vi "Wide Field Drift Correction.vi"(7 "Calling VI Ref":refnum<vi>) -> ()   [LabVIEW 2020]
uses:
  Hardware Configuration/Hardware Configuration Controls/Device Type.ctl
  Hardware Configuration/Hardware Configuration Controls/Device Function.ctl
  WFDC Controls/WFDC Notifier Element.ctl
  WFDC Controls/WFDC Actions.ctl
  <vilib>/vision/Image Controls.llb/IMAQ Image.ctl
  WFDC Controls/WFDC External Sync.ctl
  WFDC Controls/WFDC Cycle Pause.ctl
  WFDC Controls/WFDC Status.ctl
  WFDC Controls/WFDC Default XY Stage Settings.ctl
  <vilib>/Utility/miscctls.llb/LVPointTypeDef.ctl
  Orca Flash Capture Manager/Orca Flash Capture Manager Controls/Orca Flash Capture Sync.ctl
  Device Library/Cameras/IDS/IDS Controls/IDS Actions.ctl
  Device Library/Cameras/IDS/IDS Controls/IDS Parameters.ctl
  Device Library/Cameras/IDS/IDS Controls/IDS Parameter List.ctl
  Device Library/Cameras/IDS/IDS Controls/IDS ROI.ctl
  Device Library/Cameras/IDS/IDS Controls/IDS IMAQ Key Info.ctl
  Device Library/Stages/Stages Controls/Stage Actions.ctl
  e645b282-29c8-4eda-9ede-5df860dd8c52.vi
panel:
  in  "Main Tab":T1(tab)
  out "Remote Start":bool
  out "Running":bool
  out "Z Drift (µm)":dbl=1.0 format="%.3g"
  out "Axis 2 Drift (Pixels)":dbl=1.0 format="%.3g"
  out "Axis 1 Drift (Pixels)":dbl=1.0 format="%.3g"
  out "Z Stage Position":dbl(graph)
  out "Z Drift Amount":dbl(graph)
  out "XY Drift Correction Active":bool
  out "Error":bool
  in  "Setup New":bool
  in  "Find Focus":bool
  in  "Smooth Points":i32=1
  in  "Smooth Z Data":bool
  in  "Z Step Correction Limit (µm)":dbl=1.0
  in  "Stage Defaults":bool
  in  "Invert Y Axis":bool
  in  "Invert X Axis":bool
  in  "Flip XY Axis":bool
  in  "Frame Accumulations":u16=20
  in  "Calibration Scan Range (µm)":dbl=1.0
  in  "Cycle Sync XY Correction":bool=TRUE
  in  "Track XY Drift":bool=TRUE
  in  "Correct XY Drift":bool=TRUE
  in  "XY Drift Threshold (pixels)":dbl=0.2
  in  "XY Drift Step (µm)":dbl=0.1
  in  "Z Position Offset (µm)":dbl
  in  "Z Drift Threshold (µm)":dbl=0.02
  in  "Correct Z Drift":bool=TRUE
  in  "Abort Capture If Error":bool=TRUE
  in  "Cycle Sync Z Correction":bool
  out "Z Stage":dbl=1.0 format="%.3g"
  out "Z Drift":dbl=1.0 format="%.3g"
  in  "CC Box Size":i32=11
  in  "Correction Limit":u8=50
  out "Correction Step":u8=1
  out "CC Fit":dbl[][](graph)
  out "CC Image":dbl[][](graph)
  in  "Abort Remote":bool
  in  "CC Cutoff":dbl=0.2
  in  "Roundness Cutoff":dbl=1.75
  out "Axis 1":dbl=1.0 format="%.3g"
  out "Axis 2":dbl=1.0 format="%.3g"
  out "XY Active":bool
  out "Z Active":bool
  out "Error Message":string
  out "Current Frame":u32=1
  in  "Capture":bool
  in  "Number of Frames":u32=1
  in  "Image Save Path":path
  in  "Exposure Time (ms)":dbl
  in  "Image Display":bool
  in  "Live Preview":bool
  in  "Quit":bool
  # "General Settings"
  # "XY Stage Settings"
  # "XY Drift Settings"
  # "Z Drift Settings"
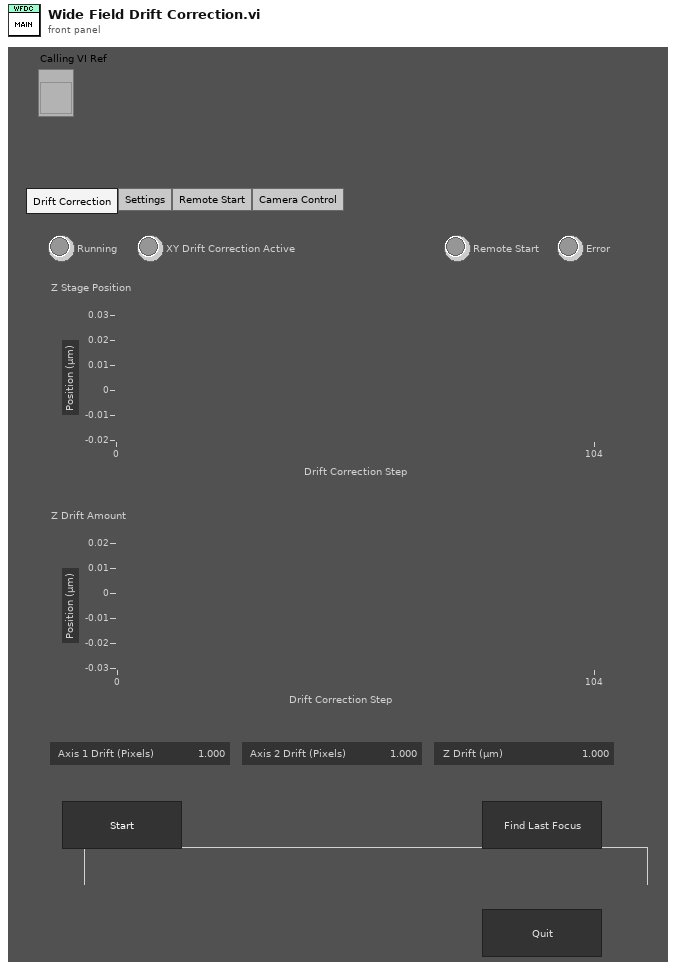
[diagram p1: front panel]
types:
  T1 = enum32{"Drift Correction", "Settings", "Remote Start", "Camera Control"}
  T2 = typedef "Orca Flash Capture Sync.ctl" = cluster{"Image Ref":T3, "Cycle Number":u16, "Camera Running?":bool, "Capture?":bool}
  T3 = typedef "IMAQ Image.ctl" = refnum<image>
  T4 = enum16{"Always On", "Always Off", "Off While Running"}
  T5 = typedef "LVPointTypeDef.ctl" = cluster{"Horizontal":i16, "Vertical":i16}
  T6 = typedef "WFDC Default XY Stage Settings.ctl" = cluster{"Flip XY":bool, "Invert X":bool, "Invert Y":bool}
  T7 = typedef "WFDC Cycle Pause.ctl" = enum16{"Pause Requested", "Paused", "Resume Requested", "Resumed"}
  T8 = typedef "WFDC Status.ctl" = enum16{"Idle", "Busy", "DC Active", "Error", "Canceled"}
  T9 = typedef "WFDC External Sync.ctl" = cluster{"Cycle Sync":T7, "Z Offset":dbl, "WFDC Status":T8}
  T10 = typedef "WFDC Actions.ctl" = enum16{"Error Check", "Remote Start", "Move to Pos", "Pre Start Get Drift", "Pre Start Check Drift", "Pre Start Z Drift", "Pre Start XY Drift", "Pre Start ReFocus", "Setup New DC", "Setup Camera", "Get Ref Images", "Calc Calibration", "Switch Tabs", "Get Drift", "Z Drift", "XY Drift", "Start Cycle", "Stop DC", "Abort Remote", "Exit Loop", "Set Error", "Generate Calibration", "Quit"}
  T11 = typedef "WFDC Notifier Element.ctl" = cluster{"WFDC Actions":T10, "Initial XYZ Positions":dbl[], "Ref Images":T3[], "Calibration (slope, inter)":dbl[], "Base Path":path, "Latest Scan Path":path, "Error":errorcluster, "XYZ Drift":dbl[]}
  T12 = typedef "Device Function.ctl" = enum16{"Primary", "Secondary", "Overview", "Wide Field Drift Correction", "642 nm Excitation", "560 nm Excitation", "940 nm Excitation", "546 nm Excitation", "488 nm Excitation", "405 nm Excitation", "Objective Drift Correction", "4Pi Objective Lock", "Objective XY", "Objective Z", "Sample XY", "Sample Coarse Z", "Sample Z", "4Pi Lower", "4Pi Upper", "Mojo", "Adj Cavity", "Line Scanning", "Alert"}
  T13 = typedef "Device Type.ctl" = enum16{"AOTF", "Camera", "Deformable Mirror", "Laser", "Microscope Base", "Shutter", "Stage", "Waveform", "FPGA", "Email", "Filter Wheel", "Spinning Disk"}
  T14 = typedef "LVRectTypeDef.ctl" = cluster{"Left":i16, "Top":i16, "Right":i16, "Bottom":i16}
  T15 = typedef "LVBoundsTypeDef.ctl" = cluster{"Width":u32, "Height":u32}
  T16 = enum8{"Enabled", "Disabled", "Disabled and Grayed Out"}
  T17 = typedef "IDS Actions.ctl" = enum16{"Error Check", "Initialize", "Preview", "Record", "Abort", "Record Settings", "Set Parameter", "Get Parameter", "Set ROI", "Get ROI", "Status", "Quit"}
  T18 = typedef "IDS Parameter List.ctl" = enum16{"Exposure Time (s)", "Binning"}
  T19 = typedef "IDS Parameters.ctl" = cluster{"Parameter":T18, "Value":dbl}
  T20 = typedef "IDS ROI.ctl" = cluster{"H Offset":i32, "V Offset":i32, "H Width":i32, "V Width":i32}
  T21 = typedef "IDS IMAQ Key Info.ctl" = cluster{"Frame":u32, "Sensor Height":i32, "Sensor Width":i32, "ROI Height":i32, "ROI Width":i32, "ROI Enable?":bool, "Bit per Pixel":u8}
  T22 = typedef "Stage Actions.ctl" = enum16{"Get Position", "MVR", "MOVE", "HALT", "ONTARGET", "ERROR", "REFERENCE", "INIT", "VELOCITY", "STATUS", "EXIT", "HOME", "ZEROPOS", "NANOPOS", "ANALOG", "QUIT"}
  T23 = enum32{"Page Enabled", "Page Disabled", "Page Disabled & Grayed"}
  T24 = typedef "2D Gaussian - Best Fit Parameters.ctl" = cluster{"Amplitude":dbl, "X Position":dbl, "Y Position":dbl, "X Width":dbl, "Y Width":dbl, "Offset":dbl}
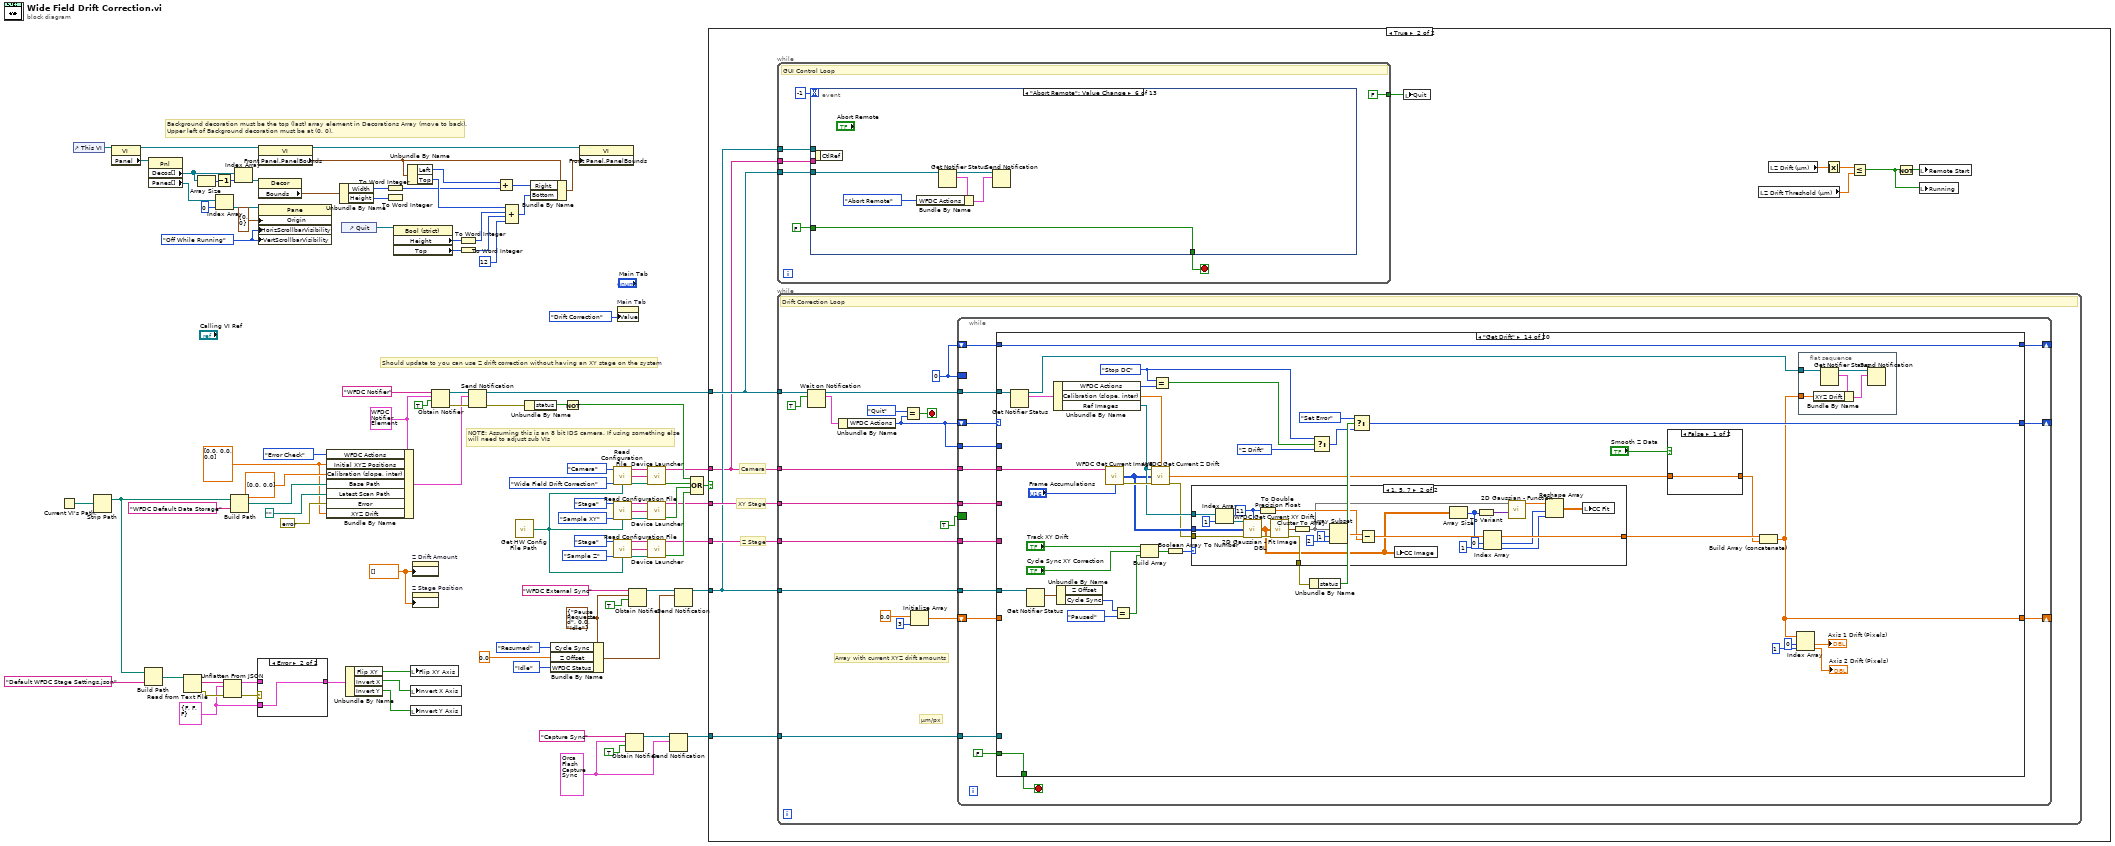
[diagram p0: block diagram]
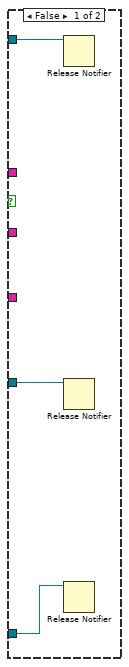
[diagram p3: hidden frame]
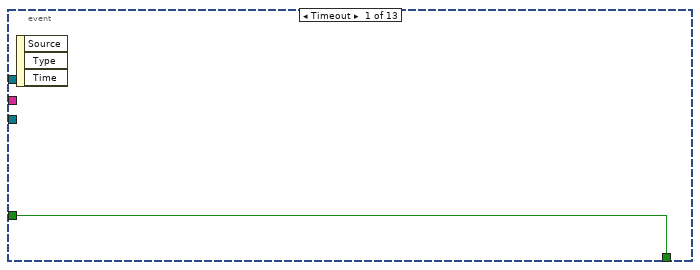
[diagram p4: hidden frame]
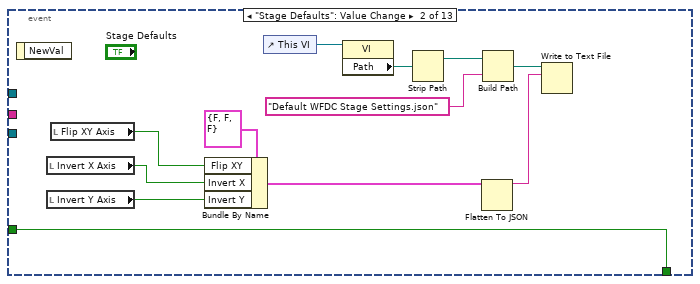
[diagram p5: hidden frame]
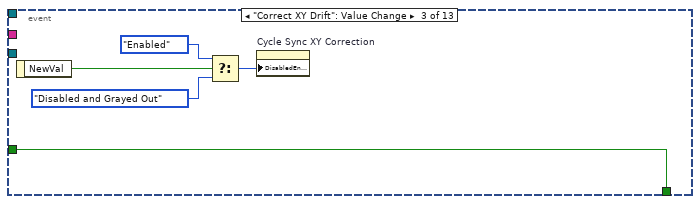
[diagram p6: hidden frame]
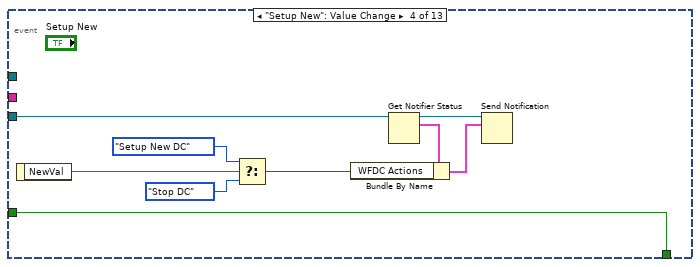
[diagram p7: hidden frame]
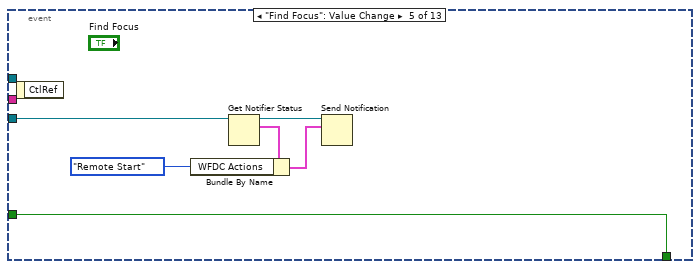
[diagram p8: hidden frame]
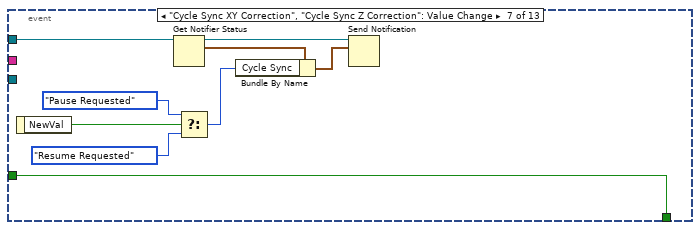
[diagram p9: hidden frame]
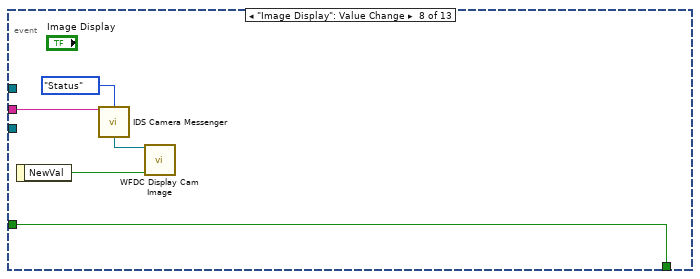
[diagram p10: hidden frame]
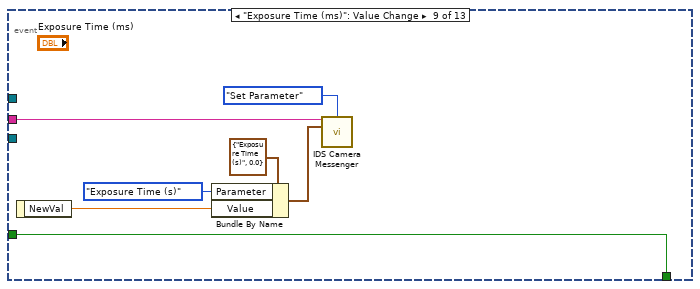
[diagram p11: hidden frame]
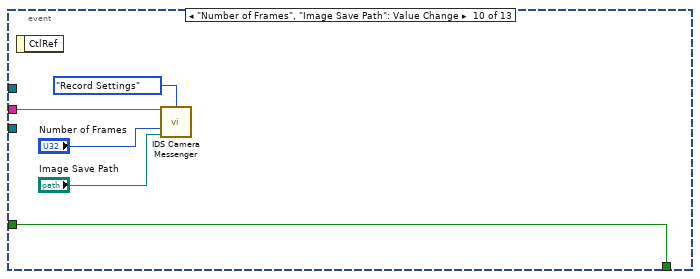
[diagram p12: hidden frame]
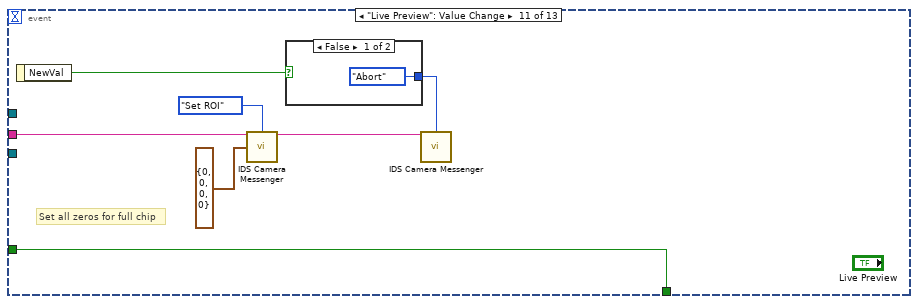
[diagram p13: hidden frame]
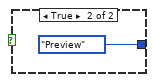
[diagram p14: hidden frame]
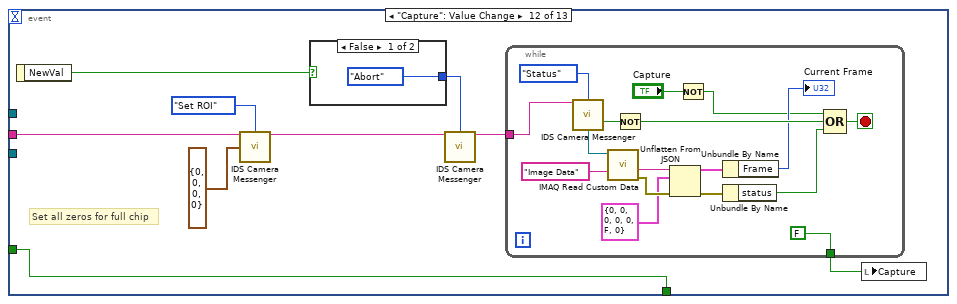
[diagram p15: hidden frame]
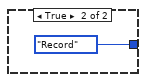
[diagram p16: hidden frame]
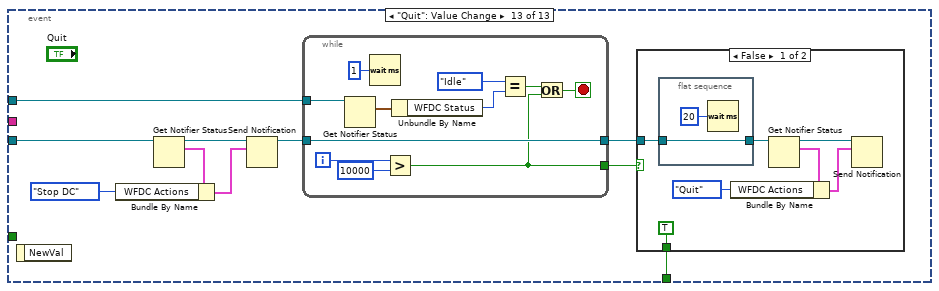
[diagram p17: hidden frame]
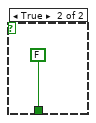
[diagram p18: hidden frame]
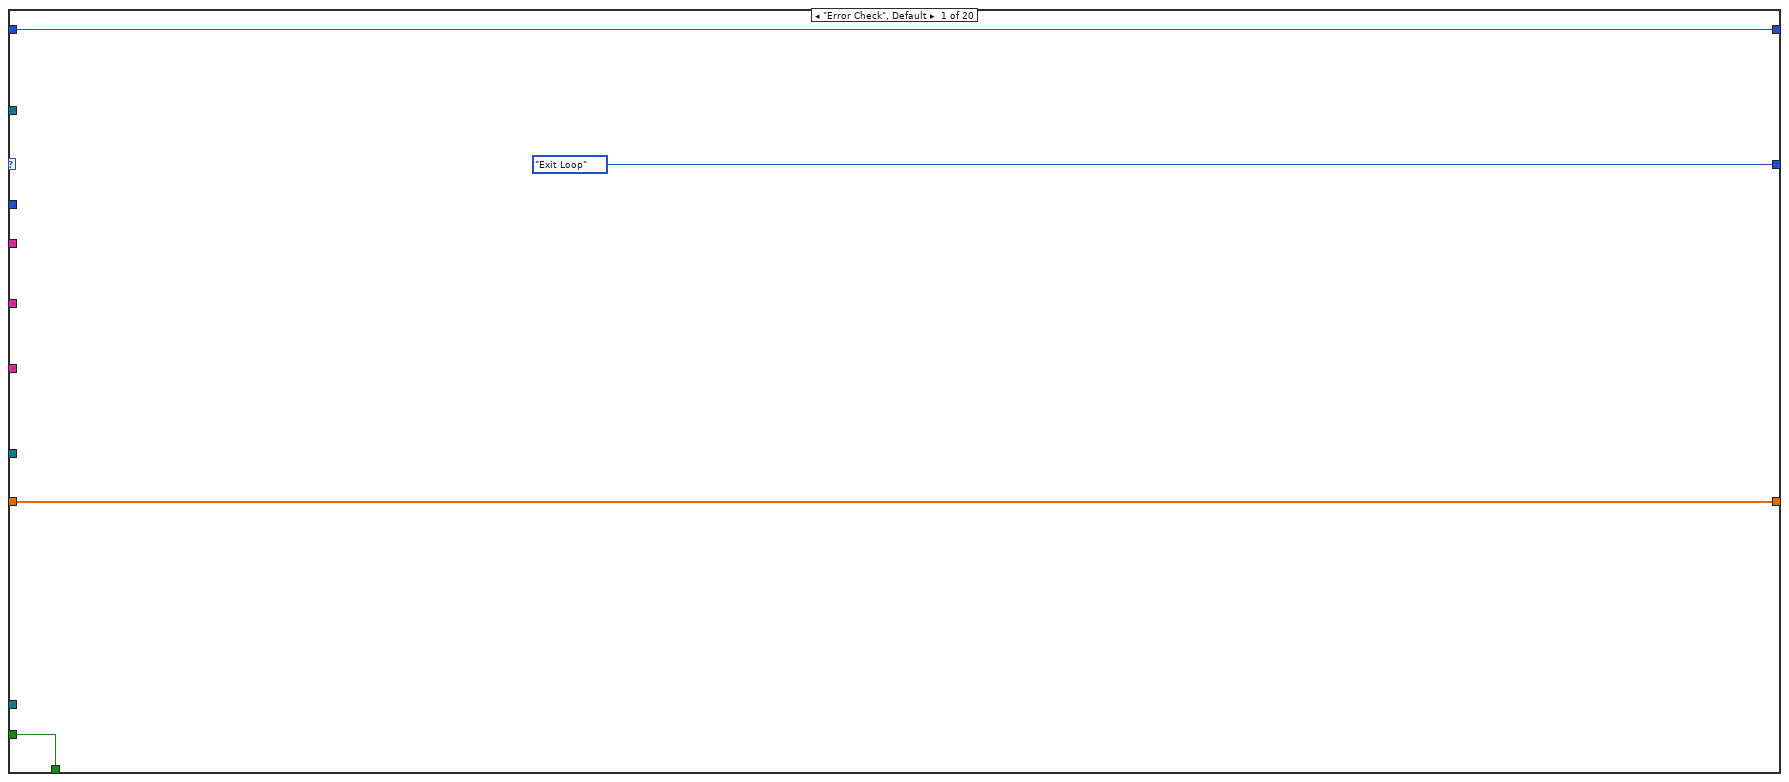
[diagram p19: hidden frame]
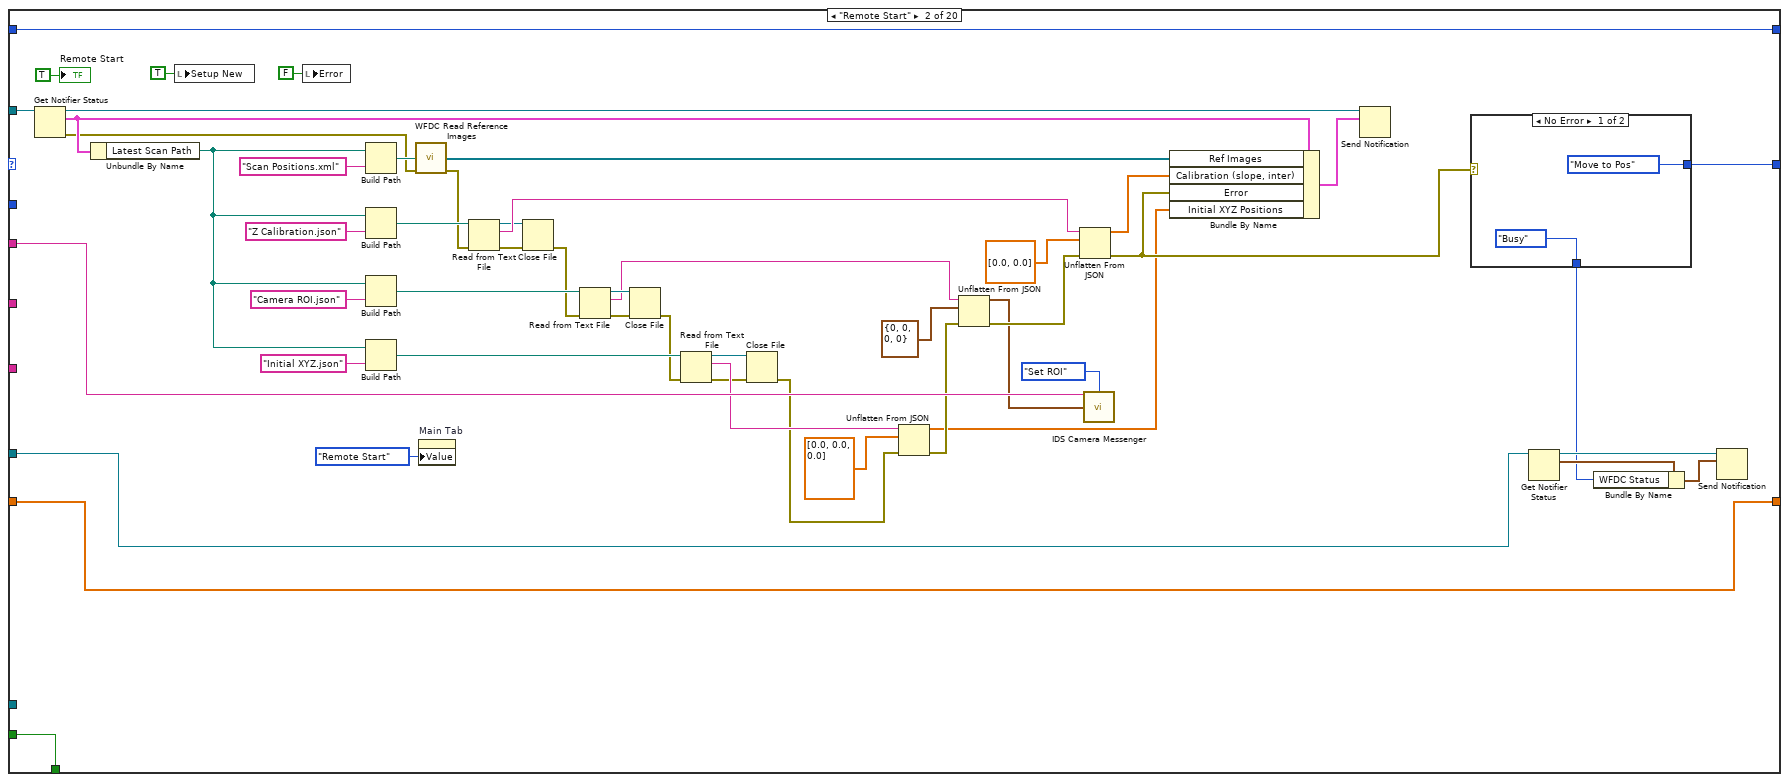
[diagram p20: hidden frame]
diagram:
  w2 = T2 {"Image Ref"=refnum, "Cycle Number"=0, "Camera Running?"=FALSE, "Capture?"=FALSE} ("Capture Sync Data")
  w17 = T4."Off While Running" ("Vertical Scrollbar Visibility")
  w39 = T6 {"Flip XY"=FALSE, "Invert X"=FALSE, "Invert Y"=FALSE} ("Default WFDC Stage Settings")
  w56 = T9 {"Cycle Sync"=enum."Pause Requested", "Z Offset"=0.0, "WFDC Status"=enum."Idle"} ("WFDC External Sync")
  w1 = dbl[] [0.0, 0.0, 0.0] ("Initial XYZ Positions")
  w65 = dbl[] []
  w67 = T11 {"WFDC Actions"=enum."Error Check", "Initial XYZ Positions"=[], "Ref Images"=[], "Calibration (slope, inter)"=[], "Base Path"=path "", "Latest Scan Path"=path "", "Error"={"status"=FALSE, "code"=0, "source"=""}, "XYZ Drift"=[]} ("WFDC Notifier Element")
  # "Background decoration must be the top (last) array element in Decorations Array (move to back).\nUpper left of Background decoration must be at (0, 0)."
  # "Should update to you can use Z drift correction without having an XY stage on the system"
  # "NOTE: Assuming this is an 8 bit IDS camera. If using something else\nwill need to adjust sub VIs"
  n1 = Current VI's Path() -> (path=w4:path)
  n2 = control-ref of="This VI"() -> (w9:refnum<vi>)
  n3 = Strip Path(path=w4) -> (stripped path=w3:path)  [unwired: 1 out]
  n4 = property class="VI"(reference=w9) -> (reference out=w18:refnum<vi>, "Panel"=w10:refnum<vi>)  [unwired: 1 in, 1 out]
  n5 = Build Path(base path=w3, name or relative path="Default WFDC Stage Settings.json") -> (appended path=w44:path)
  n6 = property class="Pnl"(reference=w10) -> ("Decos[]"=w8:refnum<vi>[], "Panes[]"=w14:refnum<vi>[])  [unwired: 1 in, 2 out]
  n7 = Read from Text File(file (use dialog)=w44) -> (text=w43:string, error out=w42:errorcluster)  [unwired: 3 in, 2 out]
  n8 = Array Size(array=w8) -> (size(s)=w6:i32)
  n9 = Decrement(x=w6) -> (x-1=w7:i32)
  n10 = Index Array(array=w14, index=0) -> (element=w13:refnum<vi>)
  n11 = Unflatten From JSON(JSON string=w43, type and defaults=w39, error in (no error)=w42) -> (value=w40:T6, error out=w41:errorcluster)  [unwired: 4 in]
  n12 = Build Path(base path=w3, name or relative path="WFDC Default Data Storage") -> (appended path=w59:path)
  n13 = Index Array(array=w8, index=w7) -> (element=w16:refnum<vi>)
  n14 = case shown="Error" w41 {
    tunnel: w40 -> [w99 _]
    tunnel: [w99 w100] -> w38
    tunnel: w39 -> [_ w100]
    frame No Error {
    }
    frame Error {
    }
  }
  n15 = property class="VI"(reference=w18) -> (reference out=w20:refnum<vi>, "Front Panel.PanelBounds"=w21:T14)  [unwired: 1 in, 1 out]
  n16 = property class="Decor"(reference=w16) -> ("Bounds"=w19:T15)  [unwired: 1 in, 2 out]
  n17 = property class="Pane"(reference=w13, "Origin"=T5 {"Horizontal"=0, "Vertical"=0}, "HorizScrollbarVisibility"=w17, "VertScrollbarVisibility"=w17) -> ()  [unwired: 1 in, 2 out]
  n18 = Bundle By Name(cluster=w67, "WFDC Actions"=WFDC_Actions."Error Check", "Initial XYZ Positions"=w1, "Calibration (slope, inter)"=dbl[] [0.0, 0.0], "Base Path"=w59, "Latest Scan Path"=path "", "Error"=errorcluster {"status"=FALSE, "code"=0, "source"=""}, "XYZ Drift"=w1) -> (w66:T11)
  n19 = Unbundle By Name(w19) -> ("Width"=w24:u32, "Height"=w27:u32)
  n20 = control-ref of="Quit"() -> (w11:refnum<vi>)
  n21 = Unbundle By Name(w38) -> ("Flip XY"=w37:bool, "Invert X"=w36:bool, "Invert Y"=w35:bool)
  n22 = To Word Integer(number=w24) -> (16bit integer=w26:i16)
  n23 = To Word Integer(number=w27) -> ()  [unwired: 1 out]
  n24 = property class="Bool (strict)"(reference=w11) -> ("Height"=w29:u32, "Top"=w30:i32)  [unwired: 1 in, 2 out]
  n25 = Unbundle By Name(w21) -> ("Left"=w23:i16, "Top"=w34:i16)
  n26 = local write "Flip XY Axis"(w37) -> ()
  n27 = local write "Invert X Axis"(w36) -> ()
  n28 = local write "Invert Y Axis"(w35) -> ()
  n29 = property on="Z Drift Amount" class="WFChart (strict)"("History Data"=w65) -> ()  [unwired: 2 in, 2 out]
  n30 = property on="Z Stage Position" class="WFChart (strict)"("History Data"=w65) -> ()  [unwired: 2 in, 2 out]
  n31 = Obtain Notifier(name (unnamed)="WFDC Notifier", notification data type=w67, create if not found? (T)=TRUE) -> (notifier out=w81:refnum<notifier>, error out=w79:errorcluster)  [unwired: 1 in, 1 out]
  n32 = To Word Integer(number=w29) -> (16bit integer=w32:i16)
  n33 = To Word Integer(number=w30) -> (16bit integer=w33:i16)
  n34 = Send Notification(notification=w66, notifier=w81, error in (no error)=w79) -> (notifier out=w80:refnum<notifier>, error out=w74:errorcluster)
  n35 = Add(x=w23, y=w26) -> (x+y=w25:i16)
  n36 = Compound Arithmetic op=ADD(w34, w32, w33, i16 12 ("y")) -> (w28:i16)
  n37 = call "Get HW Config File Path.vi"() -> ("File Path"=w63:path)  [unwired: 14 in, 1 out]
  n38 = Unbundle By Name(w74) -> ("status"=w73:bool)
  n39 = Bundle By Name(cluster=w21, "Right"=w25, "Bottom"=w28) -> (w22:T14)
  n40 = Bundle By Name(cluster=w56, "Cycle Sync"=WFDC_Cycle_Pause."Resumed", "Z Offset"=0.0, "WFDC Status"=WFDC_Status."Idle") -> (w50:T9)
  n41 = Not(x=w73) -> (.not. x?=w72:bool)
  n42 = property class="VI"(reference=w20, "Front Panel.PanelBounds"=w22) -> ()  [unwired: 1 in, 2 out]
  n43 = call "Read Configuration File.vi"("Device Type"=Device_Type."Camera", "Device Function"=Device_Function."Wide Field Drift Correction", "Config File Path"=w63) -> ("Unique Notifier Name"=w97:string, "Device Ports/IDs/Channels"=w96:string[], "Device Engine Path"=w95:path)  [unwired: 9 in, 1 out]
  n44 = call "Read Configuration File.vi"("Device Type"=Device_Type."Stage", "Device Function"=Device_Function."Sample XY", "Config File Path"=w63) -> ("Unique Notifier Name"=w88:string, "Device Ports/IDs/Channels"=w89:string[], "Device Engine Path"=w90:path)  [unwired: 9 in, 1 out]
  n45 = call "Read Configuration File.vi"("Device Type"=Device_Type."Stage", "Device Function"=Device_Function."Sample Z", "Config File Path"=w63) -> ("Unique Notifier Name"=w87:string, "Device Ports/IDs/Channels"=w86:string[], "Device Engine Path"=w85:path)  [unwired: 9 in, 1 out]
  n46 = property on="Main Tab" class="TabCtl (strict)"("Value"=T1."Drift Correction" ("Main Tab")) -> ()  [unwired: 2 in, 2 out]
  n47 = Obtain Notifier(name (unnamed)="Capture Sync", notification data type=w2, create if not found? (T)=TRUE) -> (notifier out=w47:refnum<notifier>)  [unwired: 1 in, 2 out]
  n48 = Obtain Notifier(name (unnamed)="WFDC External Sync", notification data type=w56, create if not found? (T)=TRUE) -> (notifier out=w52:refnum<notifier>)  [unwired: 1 in, 2 out]
  n49 = call "Device Launcher.vi"("Notifier Name"=w97, "Device Ports/IDs/Channels"=w96, "Device Engine Path"=w95) -> ("Notifier Name"=w70:string, "Running?"=w77:bool)  [unwired: 11 in]
  n50 = call "Device Launcher.vi"("Notifier Name"=w88, "Device Ports/IDs/Channels"=w89, "Device Engine Path"=w90) -> ("Notifier Name"=w69:string, "Running?"=w76:bool)  [unwired: 11 in]
  n51 = call "Device Launcher.vi"("Notifier Name"=w87, "Device Ports/IDs/Channels"=w86, "Device Engine Path"=w85) -> ("Notifier Name"=w68:string, "Running?"=w75:bool)  [unwired: 11 in]
  n52 = Send Notification(notification=w2, notifier=w47) -> (notifier out=w46:refnum<notifier>)  [unwired: 1 in, 1 out]
  n53 = Send Notification(notification=w50, notifier=w52) -> (notifier out=w51:refnum<notifier>)  [unwired: 1 in, 1 out]
  n54 = Compound Arithmetic op=OR(w72, w77, w76, w75) -> (w71:bool)
  n55 = case shown="True" w71 {
    tunnel: w80 -> [w103 w113]
    tunnel: w70 -> [_ w109]
    tunnel: w69 -> [_ w115]
    tunnel: w68 -> [_ w114]
    tunnel: w51 -> [w102 w111]
    tunnel: w46 -> [w101 w110]
    frame False {
      n56 = Release Notifier(notifier=w103) -> ()  [unwired: 2 in, 3 out]
      n57 = Release Notifier(notifier=w102) -> ()  [unwired: 2 in, 3 out]
      n58 = Release Notifier(notifier=w101) -> ()  [unwired: 2 in, 3 out]
    }
    frame True {
      # "Z Stage"
      # "XY Stage"
      # "Camera"
      n59 = while {
        tunnel: w113 -> [w272]
        tunnel: w109 -> [w264]
        tunnel: w115 -> [w267]
        tunnel: w114 -> [w266]
        tunnel: w111 -> [w259]
        tunnel: w110 -> [w258]
        stop <- w268 stop-if-true
        w256 = u8 0
        # "µm/px"
        # "Array with current XYZ drift amounts"
        # "Drift Correction Loop"
        n60 = Wait on Notification(notifier=w272, ignore previous (F)=TRUE) -> (notifier out=w271:refnum<notifier>, notification=w270:T11)  [unwired: 2 in, 2 out]
        n61 = Unbundle By Name(w270) -> ("WFDC Actions"=w265:T10)
        n62 = Equal?(x=WFDC_Actions."Quit", y=w265) -> (x = y?=w268:bool)
        n63 = Initialize Array(0.0 ("element"), 3 ("dimension size")) -> (w262:dbl[])
        n64 = while {
          tunnel: w271 -> [w279]
          shift-right: [w283] -> _
          shift-left: w265 -> [w287]
          tunnel: w264 -> [w286]
          tunnel: w267 -> [w285]
          tunnel: w266 -> [w284]
          tunnel: w265 -> [w280]
          tunnel: w259 -> [w278]
          shift-right: [w276] -> _
          shift-left: w262 -> [w277]
          tunnel: w258 -> [w275]
          border: TRUE -> [_]
          border: w256 -> [_]
          shift-right: [w273] -> _
          shift-left: w256 -> [w274]
          stop <- w281 stop-if-true
          n65 = case shown="\"Get Drift\"" w287 {
            selector: w287 -> [_ _ _ _ _ _ _ _ _ _ _ _ _ _ _ _ _ w1001 _ _]
            tunnel: w286 -> [_ w327 w373 w421 _ _ _ w577 _ w662 w706 w737 _ w813 _ _ _ w1013 _ _]
            tunnel: w285 -> [_ _ w360 _ _ _ w559 _ _ _ w699 _ _ _ _ w913 _ _ _ _]
            tunnel: w284 -> [_ _ w372 _ _ w484 _ w576 _ _ w696 _ _ _ w863 _ _ _ _ _]
            tunnel: [WFDC_Actions."Exit Loop" ("x") w321 WFDC_Actions."Pre Start Get Drift" ("f") w409 w454 w486 w556 w581 w641 w670 WFDC_Actions."Calc Calibration" ("x") w712 WFDC_Actions."Get Drift" ("x") w788 w852 w905 WFDC_Actions."Get Drift" ("x") WFDC_Actions."Exit Loop" ("x") WFDC_Actions."Exit Loop" ("x") WFDC_Actions."Quit" ("x")] -> w283
            tunnel: FALSE -> [w291 w343 w375 w423 w473 w489 w560 w585 w642 w672 w707 w741 w769 w815 w884 w914 w965 w1014 _ _]
            tunnel: [w291 w343 w375 w423 w473 w489 w560 w585 w642 w672 w707 w741 w769 w815 w884 w914 w965 w1014 TRUE TRUE] -> w281
            tunnel: w280 -> [_ _ _ _ _ _ _ _ w634 _ _ w714 _ _ _ _ _ _ _ _]
            tunnel: w279 -> [_ w342 w368 w422 _ w487 _ w579 _ w666 w705 w740 _ w814 w885 _ _ w1010 _ w1028]
            tunnel: w278 -> [_ w312 w353 _ _ _ _ _ w636 w658 _ w727 w758 w811 w867 w907 w963 w1003 _ w1027]
            tunnel: w277 -> [w289 w313 w369 _ w464 w477 w558 w575 w640 w668 w686 w735 w776 _ w870 w899 w966 w1008 w1019 w1026]
            tunnel: [w289 w313 w369 w408 w464 w477 w558 w575 w640 w668 w686 w735 w776 w778 w870 w899 w966 w1008 w1019 w1026] -> w276
            tunnel: w275 -> [_ _ _ _ _ _ _ _ _ _ _ _ _ _ _ _ w962 _ _ w1023]
            tunnel: w274 -> [w288 w292 w348 w379 w451 w474 w523 _ w631 w656 w678 w708 w756 w781 w851 w897 w959 w989 w1017 w1022]
            tunnel: [w288 w292 w348 w379 w450 w474 w523 u8 0 w631 w656 w678 w708 w756 w781 w851 w897 w959 w989 w1017 w1022] -> w273
            frame "Error Check", Default {
            }
            frame "Remote Start" {
              n66 = Get Notifier Status(notifier=w342) -> (notifier out=w334:refnum<notifier>, current notification=w337:T11, error out=w322:errorcluster)  [unwired: 1 in, 2 out]
              n67 = Unbundle By Name(w337) -> ("Latest Scan Path"=w314:path)
              n68 = local write "Setup New"(TRUE ("Setup New")) -> ()
              n69 = local write "Error"(FALSE ("Error")) -> ()
              n70 = Build Path(base path=w314, name or relative path="Scan Positions.xml") -> (appended path=w340:path)
              n71 = Build Path(base path=w314, name or relative path="Z Calibration.json") -> (appended path=w333:path)
              n72 = Build Path(base path=w314, name or relative path="Camera ROI.json") -> (appended path=w325:path)
              n73 = Build Path(base path=w314, name or relative path="Initial XYZ.json") -> (appended path=w311:path)
              n74 = call "WFDC Read Reference Images.vi"("Scan Positions File Path"=w340, "Error"=w322) -> ("Ref Images"=w336:T3[], "Error"=w329:errorcluster)  [unwired: 12 in]
              n75 = property on="Main Tab" class="TabCtl (strict)"("Value"=T1."Remote Start" ("Main Tab")) -> ()  [unwired: 2 in, 2 out]
              n76 = Read from Text File(file (use dialog)=w333, error in=w329) -> (refnum out=w308:refnum<file>, text=w332:string, error out=w304:errorcluster)  [unwired: 2 in, 1 out]
              n77 = Close File(refnum=w308, error in=w304) -> (error out=w301:errorcluster)  [unwired: 1 out]
              n78 = Read from Text File(file (use dialog)=w325, error in=w301) -> (refnum out=w307:refnum<file>, text=w302:string, error out=w303:errorcluster)  [unwired: 2 in, 1 out]
              n79 = Close File(refnum=w307, error in=w303) -> (error out=w298:errorcluster)  [unwired: 1 out]
              n80 = Read from Text File(file (use dialog)=w311, error in=w298) -> (refnum out=w306:refnum<file>, text=w309:string, error out=w305:errorcluster)  [unwired: 2 in, 1 out]
              n81 = Close File(refnum=w306, error in=w305) -> (error out=w299:errorcluster)  [unwired: 1 out]
              n82 = Unflatten From JSON(JSON string=w309, type and defaults=dbl[] [0.0, 0.0, 0.0], error in (no error)=w299) -> (value=w297:dbl[], error out=w300:errorcluster)  [unwired: 4 in]
              n83 = Unflatten From JSON(JSON string=w302, type and defaults=T20 {"H Offset"=0, "V Offset"=0, "H Width"=0, "V Width"=0} ("ROI Setup"), error in (no error)=w300) -> (value=w323:T20, error out=w324:errorcluster)  [unwired: 4 in]
              n84 = Unflatten From JSON(JSON string=w332, type and defaults=dbl[] [0.0, 0.0], error in (no error)=w324) -> (value=w330:dbl[], error out=w320:errorcluster)  [unwired: 4 in]
              n85 = call "IDS Camera Messenger.vi"("Notifier Name"=w327, "IDS Actions"=IDS_Actions."Set ROI", "ROI Setup"=w323) -> ()  [unwired: 7 in, 6 out]
              n86 = Bundle By Name(cluster=w337, "Ref Images"=w336, "Calibration (slope, inter)"=w330, "Error"=w320, "Initial XYZ Positions"=w297) -> (w335:T11)
              n87 = Send Notification(notification=w335, notifier=w334) -> ()  [unwired: 1 in, 2 out]
              n88 = case shown="No Error" w320 {
                tunnel: [WFDC_Actions."Move to Pos" ("x") WFDC_Actions."Exit Loop" ("x")] -> w321
                tunnel: [WFDC_Status."Busy" ("WFDC Status") WFDC_Status."Error" ("WFDC Status")] -> w317
                frame No Error {
                }
                frame Error {
                }
              }
              n89 = Get Notifier Status(notifier=w312) -> (notifier out=w319:refnum<notifier>, current notification=w318:T9)  [unwired: 1 in, 3 out]
              n90 = Bundle By Name(cluster=w318, "WFDC Status"=w317) -> (w316:T9)
              n91 = Send Notification(notification=w316, notifier=w319) -> ()  [unwired: 1 in, 2 out]
              "Remote Start" <- TRUE ("Remote Start")
            }
            frame "Move to Pos" {
              n92 = Get Notifier Status(notifier=w368) -> (current notification=w367:T11)  [unwired: 1 in, 4 out]
              n93 = Unbundle By Name(w367) -> ("Ref Images"=w366:T3[], "Initial XYZ Positions"=w359:dbl[])
              n94 = Get Notifier Status(notifier=w353) -> (notifier out=w356:refnum<notifier>, current notification=w355:T9)  [unwired: 1 in, 3 out]
              n95 = call "IDS Camera Messenger.vi"("Notifier Name"=w373, "IDS Actions"=IDS_Actions."Preview") -> ()  [unwired: 8 in, 6 out]
              n96 = Bundle By Name(cluster=w355, "WFDC Status"=WFDC_Status."Busy") -> (w354:T9)
              n97 = Split 1D Array(array=w359, index=2) -> (first subarray=w357:dbl[], second subarray=w350:dbl[])
              n98 = Send Notification(notification=w354, notifier=w356) -> ()  [unwired: 1 in, 2 out]
              n99 = Index Array(array=w366, index=1) -> ()  [unwired: 1 out]
              n100 = call "Stages Messenger.vi"("Stage Notifier Name"=w360, "Actions"=Stage_Actions."MOVE", "Setpoint"=w357, "Axis"=bool[] [TRUE, TRUE], "Exit While Busy?"=FALSE) -> ()  [unwired: 7 in, 4 out]
              n101 = call "Stages Messenger.vi"("Stage Notifier Name"=w372, "Actions"=Stage_Actions."MOVE", "Setpoint"=w350, "Axis"=bool[] [TRUE], "Exit While Busy?"=FALSE) -> ("Stage Notifier Name (Dup)"=w352:string)  [unwired: 7 in, 3 out]
              n102 = flat-sequence {
                tunnel: w352 -> [w377]
                tunnel: [w377] -> _
                frame #0 {
                  n103 = Wait (ms)(milliseconds to wait=u32 350) -> ()  [unwired: 1 out]
                }
              }
            }
            frame "Pre Start Get Drift" {
              w410 = WFDC_Actions."Abort Remote" ("x")
              n104 = Get Notifier Status(notifier=w422) -> (current notification=w420:T11)  [unwired: 1 in, 4 out]
              n105 = Unbundle By Name(w420) -> ("WFDC Actions"=w415:T10, "Initial XYZ Positions"=w378:dbl[], "Calibration (slope, inter)"=w385:dbl[], "Ref Images"=w418:T3[])
              n106 = call "WFDC Get Current Image.vi"("IDS Camera Notifier Name"=w421, "Frames"=u16 10) -> ("Image - U16"=w417:u16[][], "Error"=w419:errorcluster)  [unwired: 11 in, 1 out]
              n107 = call "WFDC Get Current Z Drift.vi"("Ref Images"=w418, "Z Calibration (slope, inter)"=w385, "Current Image"=w417, "Error In"=w419) -> ("Z Position (µm)"=w384:dbl, "Error Out"=w416:errorcluster)  [unwired: 10 in]
              n108 = Index Array(array=w418, index=1) -> (element=w403:T3)
              n109 = Index Array(array=w378, index=2) -> (element=w386:dbl)
              n110 = Subtract(x=w386, y=w384) -> (x-y=w383:dbl)
              n111 = feedback #1() -> (w394:bool)
              n112 = Select(t=35 ("hBox"), s=w394, f="CC Box Size") -> (s? t:f=w396:i32)
              n113 = call "WFDC Get Current XY Drift.vi"("Center Ref Image"=w403, "hBox"=w396, "Current Image"=w417, "Error In"=w416) -> ("Drift (px)"=w393:dbl[], "Corr Array"=w392:dbl[][], "Error Out"=w395:errorcluster)  [unwired: 9 in]
              "CC Image" <- w392
              n114 = Absolute Value(x=w393) -> (abs(x)=w381:dbl[])
              n115 = Greater?(x=w381, y=5.0) -> (0:w399:bool[])
              n116 = Or Array Elements(Boolean array=w399) -> (logical OR=w398:bool)
              n117 = feedback-in #1(w398) -> ()
              n118 = case shown="True" w394 {
                tunnel: w393 -> [_ w447]
                tunnel: w392 -> [w426 w449]
                tunnel: [w427 w446] -> w390
                tunnel: [w442 w449] -> w391
                tunnel: w395 -> [w434 w448]
                tunnel: [w431 w448] -> w389
                tunnel: w396 -> [w429 _]
                frame False {
                  n119 = To Double Precision Float(number=w429) -> (double precision float=w428:dbl)
                  n120 = Array Size(array=w426) -> (size(s)=w439:i32[])
                  n121 = call "2D Gaussian - Fit Image DBL.vi"("Image In (DBL)"=w426, "Error In"=w434) -> ("Best Fit Params"=w445:T24, "Error Out"=w433:errorcluster)  [unwired: 12 in]
                  n122 = To Variant(anything=w439) -> (Variant=w441:variant)
                  n123 = Cluster To Array(cluster=w445) -> (array=w432:dbl[])
                  n124 = Index Array(array=w439, index #1=0 ("index"), index #2=1 ("index")) -> (element #1=w438:i32, element #2=w437:i32)
                  n125 = call "2D Gaussian - Function.vi"("data"=w441, "a"=w432) -> ("f(X,a)"=w440:dbl[])  [unwired: 2 in, 2 out]
                  n126 = call "WFDC Check CC Errors.vi"("Fit Result"=w432, "CC Image"=w426, "Contrast Limit"="CC Cutoff", "Roundness Limit"="Roundness Cutoff", "Error In"=w433) -> ("Error Out"=w431:errorcluster)  [unwired: 10 in]
                  n127 = Array Subset(array=w432, index=1, length=2) -> (w430:dbl[])
                  n128 = Reshape Array(w440, w438, w437) -> (w442:dbl[][])
                  n129 = Subtract(x=w430, y=w428) -> (x-y=w427:dbl[])
                }
                frame True {
                  n130 = Reverse 1D Array(array=w447) -> (reversed array=w446:dbl[])
                }
              }
              "CC Fit" <- w391
              n131 = Unbundle By Name(w389) -> ("source"=→"Error Message":string, "status"=w388:bool)
              n132 = Build Array (concatenate)(w390, w383) -> (w408:dbl[])
              n133 = Index Array(array=w408, index #1=0 ("index"), index #2=1 ("index")) -> (element #1=→"Axis 1":dbl, element #2=→"Axis 2":dbl)
              n134 = Equal?(x=w410, y=w415) -> (x = y?=w412:bool)
              n135 = Select(t=w410, s=w412, f=WFDC_Actions."Pre Start Check Drift" ("x")) -> (s? t:f=w411:T10)
              n136 = Select(t=WFDC_Actions."Set Error" ("x"), s=w388, f=w411) -> (s? t:f=w409:T10)
            }
            frame "Pre Start Check Drift" {
              n137 = Increment(x=w451) -> (x+1=w450:u8)
              "Correction Step" <- w450
              n138 = local read "Z Drift Threshold (µm)"() -> (w461:dbl)
              n139 = local read "XY Drift Threshold (pixels)"() -> (w466:dbl)
              n140 = Index Array(array=w464, index=2) -> (element=w462:dbl)
              n141 = Array Subset(array=w464, index=0, length=2) -> (w467:dbl[])
              n142 = Absolute Value(x=w462) -> (abs(x)=w453:dbl)
              n143 = Absolute Value(x=w467) -> (abs(x)=w452:dbl[])
              n144 = Greater?(x=w453, y=w461) -> (0:w459:bool)
              n145 = Greater?(x=w452, y=w466) -> (0:w465:bool[])
              n146 = Or Array Elements(Boolean array=w465) -> (logical OR=w460:bool)
              n147 = Or(x=w460, y=w459) -> (x .or. y?=w458:bool)
              n148 = Greater?(x=w450, y="Correction Limit") -> (0:w457:bool)
              n149 = Select(t=WFDC_Actions."Pre Start Z Drift" ("x"), s=w458, f=WFDC_Actions."Switch Tabs") -> (s? t:f=w455:T10)
              n150 = Select(t=WFDC_Actions."Pre Start ReFocus" ("f"), s=w457, f=w455) -> (s? t:f=w454:T10)
            }
            frame "Pre Start Z Drift" {
              n151 = Get Notifier Status(notifier=w487) -> (current notification=w488:T11)  [unwired: 1 in, 4 out]
              n152 = Unbundle By Name(w488) -> ("WFDC Actions"=w485:T10)
              n153 = local write "XY Active"(FALSE ("XY Active")) -> ()
              n154 = Array Subset(array=w477, index=0, length=2) -> (w482:dbl[])
              n155 = Absolute Value(x=w482) -> (abs(x)=w481:dbl[])
              n156 = Greater?(x=w481, y=5.0) -> (0:w478:bool[])
              n157 = Or Array Elements(Boolean array=w478) -> (logical OR=w476:bool)
              n158 = case shown="False" w476 {
                tunnel: [w504 WFDC_Actions."Pre Start XY Drift" ("x")] -> w486
                tunnel: w485 -> [w503 _]
                tunnel: w477 -> [w501 _]
                tunnel: w484 -> [w497 _]
                frame False {
                  w505 = WFDC_Actions."Abort Remote" ("x")
                  n159 = local read "Z Drift Threshold (µm)"() -> (w499:dbl)
                  n160 = Index Array(array=w501, index=2) -> (element=w491:dbl)
                  "Z Drift" <- w491
                  n161 = Absolute Value(x=w491) -> (abs(x)=w500:dbl)
                  n162 = Greater?(x=w500, y=w499) -> (0:w498:bool)
                  n163 = case shown="True" w498 {
                    tunnel: w497 -> [w512 w521]
                    tunnel: w491 -> [_ w518]
                    tunnel: [w510 w515] -> w496
                    tunnel: [w511 w514] -> w494
                    frame False {
                      n164 = call "Stages Messenger.vi"("Stage Notifier Name"=w512, "Actions"=Stage_Actions."Get Position") -> ("Positions"=w511:dbl[], "Error"=w510:errorcluster)  [unwired: 10 in, 2 out]
                    }
                    frame True {
                      n165 = Build Array(w518) -> (w520:dbl[])
                      n166 = call "Stages Messenger.vi"("Stage Notifier Name"=w521, "Actions"=Stage_Actions."MVR", "Setpoint"=w520, "Axis"=bool[] [TRUE], "Exit While Busy?"=FALSE) -> ("Positions"=w514:dbl[], "Error"=w515:errorcluster)  [unwired: 7 in, 2 out]
                    }
                  }
                  n167 = Unbundle By Name(w496) -> ("status"=w495:bool)
                  n168 = Index Array(array=w494, index=0) -> (element=→"Z Stage":dbl)
                  n169 = Equal?(x=w505, y=w503) -> (x = y?=w507:bool)
                  n170 = Select(t=w505, s=w507, f=WFDC_Actions."Pre Start XY Drift" ("x")) -> (s? t:f=w506:T10)
                  n171 = Select(t=WFDC_Actions."Set Error" ("x"), s=w495, f=w506) -> (s? t:f=w504:T10)
                  "Z Active" <- TRUE ("Z Active")
                }
                frame True {
                }
              }
            }
            frame "Pre Start XY Drift" {
              n172 = local read "CC Box Size"() -> (w547:i32)
              n173 = local write "Z Active"(FALSE ("Z Active")) -> ()
              n174 = Array Subset(array=w558, index=0, length=2) -> (w525:dbl[])
              n175 = To Double Precision Float(number=w547) -> (double precision float=w546:dbl)
              n176 = Absolute Value(x=w525) -> (abs(x)=w541:dbl[])
              n177 = Subtract(x=w546, y=3.0) -> ()  [unwired: 1 out]
              n178 = Greater?(x=w541, y=5.0) -> (0:w545:bool[])
              n179 = local read "Flip XY Axis"() -> (w537:bool)
              n180 = local read "XY Drift Step (µm)"() -> (w528:dbl)
              n181 = local read "XY Drift Threshold (pixels)"() -> (w531:dbl)
              n182 = Or Array Elements(Boolean array=w545) -> (logical OR=w529:bool)
              n183 = Select(t=0.5, s=w529, f=w528) -> (s? t:f=w527:dbl)
              n184 = Absolute Value(x=w525) -> (abs(x)=w532:dbl[])
              n185 = Greater?(x=w532, y=w531) -> (0:w530:bool[])
              n186 = case shown="True" w537 {
                tunnel: w530 -> [w562 w566]
                tunnel: [w562 w565] -> w550
                tunnel: w525 -> [w561 w564]
                tunnel: [w561 w563] -> w535
                frame False {
                }
                frame True {
                  n187 = Reverse 1D Array(array=w564) -> (reversed array=w563:dbl[])
                  n188 = Reverse 1D Array(array=w566) -> (reversed array=w565:bool[])
                }
              }
              n189 = Greater?(x=w535, y=0.0) -> (0:w534:bool[])
              n190 = local read "Invert X Axis"() -> (w539:bool)
              n191 = local read "Invert Y Axis"() -> (w540:bool)
              n192 = Build Array(w539, w540) -> (w538:bool[])
              n193 = for {
                N: 2 -> [_]
                tunnel: [w571] -> w549 mode=indexing
                tunnel: w527 -> [w569]
                tunnel: w538 -> [w572] mode=indexing
                tunnel: w534 -> [w567] mode=indexing
                n194 = Negate(x=w569) -> (-x=w570:dbl)
                n195 = Select(t=w569, s=w567, f=w570) -> (s? t:f=w568:dbl)
                n196 = Negate(x=w568) -> (-x=w573:dbl)
                n197 = Select(t=w568, s=w572, f=w573) -> (s? t:f=w571:dbl)
              }
              n198 = call "Stages Messenger.vi"("Stage Notifier Name"=w559, "Actions"=Stage_Actions."MVR", "Setpoint"=w549, "Axis"=w550, "Exit While Busy?"=FALSE) -> ("Error"=w544:errorcluster)  [unwired: 7 in, 3 out]
              n199 = Select(t=WFDC_Actions."Set Error" ("x"), s=w544, f=WFDC_Actions."Pre Start Get Drift" ("x")) -> (s? t:f=w556:T10)
              "XY Active" <- TRUE ("XY Active")
            }
            frame "Pre Start ReFocus" {
              n200 = Get Notifier Status(notifier=w579) -> (current notification=w580:T11)  [unwired: 1 in, 4 out]
              n201 = feedback #2() -> (w583:u8)
              n202 = Increment(x=w583) -> (x+1=w584:u8)
              n203 = feedback-in #2(w584) -> ()
              n204 = Unbundle By Name(w580) -> ("Ref Images"=w578:T3[])
              n205 = Greater Than 0?(x=w583) -> (x > 0?=w582:bool)
              n206 = case shown="False" w582 {
                tunnel: [w591 WFDC_Actions."Abort Remote" ("x")] -> w581
                tunnel: w578 -> [w599 _]
                tunnel: w577 -> [w596 _]
                tunnel: w576 -> [w590 _]
                frame False {
                  n207 = Build Array(-20.0 ("element")) -> (w595:dbl[])
                  n208 = call "Stages Messenger.vi"("Stage Notifier Name"=w590, "Actions"=Stage_Actions."MVR", "Setpoint"=w595, "Axis"=bool[] [TRUE], "Exit While Busy?"=FALSE) -> ("Stage Notifier Name (Dup)"=w588:string)  [unwired: 7 in, 3 out]
                  n209 = call "Stall Data Flow.vim"("value in"=w588, "milliseconds to wait"=u32 300) -> ("value out"=w587:string)  [unwired: 1 out]
                  n210 = Index Array(array=w599, index=1) -> (element=w597:T3)
                  n211 = call "WFDC Scan Focus.vi"("Ref Image"=w597, "Camera Notifier"=w596, "Z Stage Notifier"=w587, "No. of Steps"=40, "Step Size (µm)"=1.0) -> ("Z Stage Notifier (Dup)"=w602:string, "Pos vs. Corr"=w601:dbl[][], "Canceled?"=w600:bool)  [unwired: 8 in]
                  n212 = case shown="True" w600 {
                    tunnel: w602 -> [w607 _]
                    tunnel: w601 -> [w606 _]
                    tunnel: [WFDC_Actions."Pre Start Get Drift" ("f") WFDC_Actions."Abort Remote" ("f")] -> w591
                    frame False {
                      n213 = Index Array(array=w606, index (col) #1=0 ("disabled index (col)"), index (col) #2=1 ("index (col)")) -> (element #1=w609:dbl[], element #2=w610:dbl[])  [unwired: 2 in]
                      n214 = disable-structure shown="Enabled" {
                        disable-tunnel: w610 -> [w616 w620]
                        disable-tunnel: w609 -> [w615 w621]
                        disable-tunnel: [w613 w617] -> w608
                        frame Enabled {
                          n215 = Array Max & Min(array=w616) -> (max index (indices)=w614:i32)  [unwired: 3 out]
                          n216 = Index Array(array=w615, index=w614) -> (element=w613:dbl)
                        }
                        frame Disabled {
                          n217 = call "1D Gaussian Fitting.vi"("X Values"=w621, "Y Values"=w620) -> ("Best Fit Parameters"=w619:dbl[])  [unwired: 11 in, 2 out]
                          n218 = Index Array(array=w619, index=1) -> (element=w617:dbl)
                        }
                      }
                      n219 = flat-sequence {
                        tunnel: w607 -> [w624]
                        tunnel: w608 -> [w623]
                        frame #0 {
                          n220 = Build Array(w623) -> (w622:dbl[])
                          n221 = call "Stages Messenger.vi"("Stage Notifier Name"=w624, "Actions"=Stage_Actions."MOVE", "Setpoint"=w622, "Axis"=bool[] [TRUE], "Exit While Busy?"=FALSE) -> ()  [unwired: 7 in, 4 out]
                        }
                        frame #1 {
                          n222 = Wait (ms)(milliseconds to wait=u32 350) -> ()  [unwired: 1 out]
                        }
                      }
                    }
                    frame True {
                    }
                  }
                }
                frame True {
                }
              }
            }
            frame "Setup New DC", "Generate Calibration" {
              n223 = case shown="\"Generate Calibration\", Default" w634 {
                tunnel: [WFDC_Actions."Setup Camera" ("f") w646] -> w641
                frame "Generate Calibration", Default {
                }
                frame "Setup New DC" {
                  n224 = Two Button Dialog(message="Is the Z stage is near its center position?", 1:"No" ("F button name (\"Cancel\")"), 2:"Yes" ("T button name (\"OK\")")) -> (T button?=w649:bool)
                  n225 = case shown="False" w649 {
                    selector: w649 -> [w653 w655]
                    tunnel: "Center Z Stage and start again" ("message") -> [w654 _]
                    tunnel: [w653 w655] -> w644
                    frame False {
                      n226 = One Button Dialog(message=w654) -> ()  [unwired: 1 in, 1 out]
                    }
                    frame True {
                    }
                  }
                  n227 = Select(t=WFDC_Actions."Setup Camera" ("x"), s=w644, f=WFDC_Actions."Exit Loop") -> (s? t:f=w646:T10)
                }
              }
              n228 = Get Notifier Status(notifier=w636) -> (notifier out=w638:refnum<notifier>, current notification=w637:T9)  [unwired: 1 in, 3 out]
              n229 = Bundle By Name(cluster=w637, "WFDC Status"=WFDC_Status."Busy") -> (w639:T9)
              n230 = local write "Error"(FALSE ("Error")) -> ()
              n231 = Send Notification(notification=w639, notifier=w638) -> ()  [unwired: 1 in, 2 out]
              "Running" <- TRUE ("Running")
            }
            frame "Setup Camera" {
              w669 = dbl[] []
              # "Set exposure time and select camera ROI"
              n232 = Get Notifier Status(notifier=w666) -> (notifier out=w667:refnum<notifier>, current notification=w665:T11)  [unwired: 1 in, 3 out]
              n233 = Unbundle By Name(w665) -> ("Base Path"=w661:path)
              n234 = property on="Z Drift Amount" class="WFChart (strict)"("History Data"=w669) -> ()  [unwired: 2 in, 2 out]
              n235 = property on="Z Stage Position" class="WFChart (strict)"("History Data"=w669) -> ()  [unwired: 2 in, 2 out]
              n236 = call "WFDC Setup Camera.vi"("Base Data Path"=w661, "Camera Notifier Name"=w662, "ROI File Name"="Camera ROI.json" ("name or relative path")) -> ("Current Save Path"=w663:path, "Canceled?"=w657:bool)  [unwired: 9 in, 2 out]
              n237 = Bundle By Name(cluster=w665, "Latest Scan Path"=w663) -> (w664:T11)
              n238 = Send Notification(notification=w664, notifier=w667) -> ()  [unwired: 1 in, 2 out]
              n239 = case shown="False" w657 {
                tunnel: w658 -> [_ w673]
                frame False {
                }
                frame True {
                  n240 = Get Notifier Status(notifier=w673) -> (notifier out=w676:refnum<notifier>, current notification=w675:T9)  [unwired: 1 in, 3 out]
                  n241 = Bundle By Name(cluster=w675, "WFDC Status"=WFDC_Status."Canceled") -> (w677:T9)
                  n242 = Send Notification(notification=w677, notifier=w676) -> ()  [unwired: 1 in, 2 out]
                }
              }
              n243 = Select(t=WFDC_Actions."Exit Loop", s=w657, f=WFDC_Actions."Get Ref Images" ("y")) -> (s? t:f=w670:T10)
            }
            frame "Get Ref Images" {
              n244 = call "Stages Messenger.vi"("Stage Notifier Name"=w699, "Actions"=Stage_Actions."Get Position") -> ("Positions"=w691:dbl[])  [unwired: 10 in, 3 out]
              n245 = call "Stages Messenger.vi"("Stage Notifier Name"=w696, "Actions"=Stage_Actions."Get Position") -> ("Stage Notifier Name (Dup)"=w695:string, "Positions"=w694:dbl[])  [unwired: 10 in, 2 out]
              n246 = Index Array(array=w691, index #1=0 ("index"), index #2=1 ("index")) -> (element #1=w689:dbl, element #2=w688:dbl)
              n247 = Index Array(array=w694, index=0) -> (element=w687:dbl)
              n248 = Get Notifier Status(notifier=w705) -> (notifier out=w703:refnum<notifier>, current notification=w702:T11)  [unwired: 1 in, 3 out]
              n249 = Unbundle By Name(w702) -> ("Latest Scan Path"=w682:path)
              n250 = Build Array(w689, w688, w687) -> (w683:dbl[])
              n251 = call "WFDC Get Reference Images.vi"("IDS Camera Notifier"=w706, "Data Save Path"=w682, "Z Stage Notifier"=w695, "Scan Range"="Calibration Scan Range (µm)", "Frame per Step"=u32 20, "Scan Positions File Name"="Scan Positions.xml" ("name or relative path")) -> ()  [unwired: 10 in]
              n252 = Build Path(base path=w682, name or relative path="Initial XYZ.json") -> (appended path=w680:path)
              n253 = Flatten To JSON(anything=w683) -> (JSON string=w679:string)  [unwired: 2 in, 1 out]
              n254 = Bundle By Name(cluster=w702, "Initial XYZ Positions"=w683) -> (w701:T11)
              n255 = Write to Text File(file (use dialog)=w680, text=w679) -> ()  [unwired: 2 in, 3 out]
              n256 = Send Notification(notification=w701, notifier=w703) -> ()  [unwired: 1 in, 2 out]
            }
            frame "Calc Calibration" {
              n257 = local read "Cycle Sync XY Correction"() -> (w726:bool)
              n258 = local read "Cycle Sync Z Correction"() -> (w725:bool)
              n259 = Get Notifier Status(notifier=w740) -> (notifier out=w711:refnum<notifier>, current notification=w739:T11)  [unwired: 1 in, 3 out]
              n260 = flat-sequence {
                tunnel: w739 -> [w755]
                tunnel: [w753] -> w738
                tunnel: w737 -> [w750]
                tunnel: [w750] -> w736
                tunnel: [w748] -> w728
                tunnel: w727 -> [w748]
                tunnel: [w746] -> w722
                tunnel: [w745] -> w723
                tunnel: w716 -> [w744]
                frame #0 {
                  n261 = Unbundle By Name(w755) -> ("Latest Scan Path"=w746:path)
                  n262 = call "WFDC Compute Z Calibration.vi"("Scan Positions File Name"="Scan Positions.xml" ("name or relative path"), "User Close?"=w744, "Data Path"=w746) -> ("Fit Slope"=w754:dbl, "Fit Intercept"=w752:dbl, "Ref Images"=w749:T3[], "Error"=w751:errorcluster)  [unwired: 9 in]
                  n263 = Build Array(w754, w752) -> (w745:dbl[])
                  n264 = Bundle By Name(cluster=w755, "Calibration (slope, inter)"=w745, "Error"=w751, "Ref Images"=w749) -> (w753:T11)
                }
              }
              n265 = Or(x=w726, y=w725) -> (x .or. y?=w724:bool)
              n266 = Equal?(x=WFDC_Actions."Generate Calibration", y=w714) -> (x = y?=w710:bool)
              n267 = Equal?(x=WFDC_Actions."Setup New DC", y=w714) -> (x = y?=w716:bool)
              n268 = Select(t=WFDC_Cycle_Pause."Pause Requested" ("Cycle Sync"), s=w724, f=WFDC_Cycle_Pause."Resumed" ("Cycle Sync")) -> (s? t:f=w730:T7)
              n269 = Get Notifier Status(notifier=w728) -> (notifier out=w734:refnum<notifier>, current notification=w733:T9)  [unwired: 1 in, 3 out]
              n270 = Bundle By Name(cluster=w733, "Cycle Sync"=w730) -> (w732:T9)
              n271 = Send Notification(notification=w732, notifier=w734) -> ()  [unwired: 1 in, 2 out]
              n272 = Send Notification(notification=w738, notifier=w711) -> ()  [unwired: 1 in, 2 out]
              n273 = Flatten To JSON(anything=w723) -> (JSON string=w719:string)  [unwired: 2 in, 1 out]
              n274 = Build Path(base path=w722, name or relative path="Z Calibration.json") -> (appended path=w720:path)
              n275 = Write to Text File(file (use dialog)=w720, text=w719) -> (refnum out=w718:refnum<file>)  [unwired: 2 in, 2 out]
              n276 = Close File(refnum=w718) -> ()  [unwired: 1 in, 2 out]
              n277 = case shown="True" w710 {
                tunnel: w736 -> [w743 _]
                frame False {
                  # "Start Camera"
                  n278 = call "IDS Camera Messenger.vi"("Notifier Name"=w743, "IDS Actions"=IDS_Actions."Preview") -> ()  [unwired: 8 in, 6 out]
                }
                frame True {
                }
              }
              n279 = Select(t=WFDC_Actions."Stop DC", s=w710, f=WFDC_Actions."Switch Tabs" ("x")) -> (s? t:f=w712:T10)
            }
            frame "Switch Tabs" {
              w757 = FALSE ("Z Active")
              n280 = local read "Cycle Sync XY Correction"() -> (w768:bool)
              n281 = local read "Cycle Sync Z Correction"() -> (w767:bool)
              n282 = local write "Z Active"(w757) -> ()
              n283 = local write "XY Active"(w757) -> ()
              n284 = local write "Remote Start"(w757) -> ()
              n285 = property on="Main Tab" class="TabCtl (strict)"("Value"=T1."Drift Correction" ("Main Tab")) -> ("Pages"=w773:refnum<vi>[])  [unwired: 2 in, 2 out]
              n286 = Or(x=w768, y=w767) -> (x .or. y?=w766:bool)
              n287 = Index Array(array=w773, index=3) -> (element=w771:refnum<vi>)
              n288 = property class="Page"(reference=w771, "PageEnb"=T23."Page Disabled & Grayed" ("Page Enabled State")) -> ()  [unwired: 1 in, 2 out]
              n289 = Select(t=WFDC_Cycle_Pause."Pause Requested" ("Cycle Sync"), s=w766, f=WFDC_Cycle_Pause."Resume Requested" ("Cycle Sync")) -> (s? t:f=w765:T7)
              n290 = Get Notifier Status(notifier=w758) -> (notifier out=w762:refnum<notifier>, current notification=w763:T9)  [unwired: 1 in, 3 out]
              n291 = Bundle By Name(cluster=w763, "WFDC Status"=WFDC_Status."DC Active", "Cycle Sync"=w765) -> (w764:T9)
              n292 = Send Notification(notification=w764, notifier=w762) -> ()  [unwired: 1 in, 2 out]
            }
            frame "Get Drift" {
              w789 = WFDC_Actions."Stop DC" ("x")
              n293 = Get Notifier Status(notifier=w814) -> (notifier out=w777:refnum<notifier>, current notification=w779:T11)  [unwired: 1 in, 3 out]
              n294 = Get Notifier Status(notifier=w811) -> (current notification=w810:T9)  [unwired: 1 in, 4 out]
              n295 = Unbundle By Name(w779) -> ("WFDC Actions"=w795:T10, "Calibration (slope, inter)"=w807:dbl[], "Ref Images"=w800:T3[])
              n296 = Unbundle By Name(w810) -> ("Cycle Sync"=w808:T7)  [unwired: 1 out]
              n297 = call "WFDC Get Current Image.vi"("IDS Camera Notifier Name"=w813, "Frames"="Frame Accumulations") -> ("Image - U16"=w799:u16[][], "Error"=w806:errorcluster)  [unwired: 11 in, 1 out]
              n298 = Equal?(x=w808, y=WFDC_Cycle_Pause."Paused") -> (x = y?=w803:bool)
              n299 = Build Array("Track XY Drift", "Cycle Sync XY Correction", w803) -> (w802:bool[])
              n300 = call "WFDC Get Current Z Drift.vi"("Ref Images"=w800, "Z Calibration (slope, inter)"=w807, "Current Image"=w799, "Error In"=w806) -> ("Z Position (µm)"=w783:dbl, "Error Out"=w798:errorcluster)  [unwired: 10 in]
              n301 = Equal?(x=w789, y=w795) -> (x = y?=w791:bool)
              n302 = Boolean Array To Number(Boolean array=w802) -> (number=w801:u8)
              n303 = case shown="1, 5, 7" w801 {
                tunnel: w800 -> [_ w850]
                tunnel: w799 -> [_ w847]
                tunnel: w798 -> [w826 w846]
                tunnel: [dbl[] [0.0, 0.0] w838] -> w797
                tunnel: [w826 w837] -> w796
                frame 0, 2..4, 6, Default {
                }
                frame 1, 5, 7 {
                  w839 = 11 ("hBox")
                  n304 = Index Array(array=w850, index=1) -> (element=w848:T3)
                  n305 = call "WFDC Get Current XY Drift.vi"("Center Ref Image"=w848, "hBox"=w839, "Current Image"=w847, "Error In"=w846) -> ("Corr Array"=w829:dbl[][], "Error Out"=w840:errorcluster)  [unwired: 9 in, 1 out]
                  n306 = To Double Precision Float(number=w839) -> (double precision float=w843:dbl)
                  n307 = call "2D Gaussian - Fit Image DBL.vi"("Image In (DBL)"=w829, "Error In"=w840) -> ("Best Fit Params"=w845:T24, "Error Out"=w837:errorcluster)  [unwired: 12 in]
                  n308 = Cluster To Array(cluster=w845) -> (array=w828:dbl[])
                  n309 = Array Subset(array=w828, index=1, length=2) -> (w844:dbl[])
                  n310 = Subtract(x=w844, y=w843) -> (x-y=w838:dbl[])
                  n311 = local write "CC Image"(w829) -> ()
                  n312 = Array Size(array=w829) -> (size(s)=w834:i32[])
                  n313 = To Variant(anything=w834) -> (Variant=w832:variant)
                  n314 = Index Array(array=w834, index #1=0 ("index"), index #2=1 ("index")) -> (element #1=w835:i32, element #2=w836:i32)
                  n315 = call "2D Gaussian - Function.vi"("data"=w832, "a"=w828) -> ("f(X,a)"=w833:dbl[])  [unwired: 2 in, 2 out]
                  n316 = Reshape Array(w833, w835, w836) -> (w827:dbl[][])
                  n317 = local write "CC Fit"(w827) -> ()
                }
              }
              n318 = Unbundle By Name(w796) -> ("status"=w794:bool)
              n319 = Select(t=w789, s=w791, f=WFDC_Actions."Z Drift" ("x")) -> (s? t:f=w790:T10)
              n320 = Select(t=WFDC_Actions."Set Error" ("x"), s=w794, f=w790) -> (s? t:f=w788:T10)
              n321 = case shown="False" "Smooth Z Data" {
                tunnel: w783 -> [w821 w824]
                tunnel: [w821 w823] -> w782
                frame False {
                }
                frame True {
                  n322 = call "Rolling Average.vi"("Smooth Pts"="Smooth Points", "Input"=w824) -> ("Output"=w823:dbl)  [unwired: 13 in]
                }
              }
              n323 = Build Array (concatenate)(w797, w782) -> (w778:dbl[])
              n324 = Index Array(array=w778, index #1=0 ("index"), index #2=1 ("index")) -> (element #1=→"Axis 1 Drift (Pixels)":dbl, element #2=→"Axis 2 Drift (Pixels)":dbl)
              n325 = flat-sequence {
                tunnel: w778 -> [w820]
                tunnel: w777 -> [w816]
                frame #0 {
                  n326 = Get Notifier Status(notifier=w816) -> (notifier out=w818:refnum<notifier>, current notification=w817:T11)  [unwired: 1 in, 3 out]
                  n327 = Bundle By Name(cluster=w817, "XYZ Drift"=w820) -> (w819:T11)
                  n328 = Send Notification(notification=w819, notifier=w818) -> ()  [unwired: 1 in, 2 out]
                }
              }
            }
            frame "Z Drift" {
              # "Z Pos"
              # "Initial Z Position"
              n329 = Get Notifier Status(notifier=w885) -> (current notification=w886:T11)  [unwired: 1 in, 4 out]
              n330 = Get Notifier Status(notifier=w867) -> (current notification=w859:T9)  [unwired: 1 in, 4 out]
              n331 = Unbundle By Name(w886) -> ("Initial XYZ Positions"=w871:dbl[])
              n332 = Unbundle By Name(w859) -> ("Z Offset"=w858:dbl, "Cycle Sync"=w864:T7)
              n333 = Equal?(x=WFDC_Cycle_Pause."Paused" ("y"), y=w864) -> (x = y?=w861:bool)
              n334 = Index Array(array=w871, index=2) -> (element=w883:dbl)
              n335 = Index Array(array=w870, index=2) -> (element=w868:dbl)
              n336 = Select(t=w861, s="Cycle Sync Z Correction", f=TRUE) -> (s? t:f=w860:bool)
              n337 = Compound Arithmetic op=ADD("Z Position Offset (µm)", w883, w858) -> (w882:dbl)
              n338 = Subtract(x=w882, y=w868) -> (x-y=w857:dbl)
              "Z Drift Amount" <- w857
              "Z Drift (µm)" <- w857
              n339 = Absolute Value(x=w857) -> (abs(x)=w877:dbl)
              n340 = Greater?(x=w877, y="Z Drift Threshold (µm)") -> (0:w876:bool)
              n341 = Less Or Equal?(x=w857, y="Z Step Correction Limit (µm)") -> (x <= y?=w855:bool)
              n342 = Compound Arithmetic op=AND(w855, w876, "Correct Z Drift", w860) -> (w874:bool)
              n343 = case shown="True" w874 {
                tunnel: w863 -> [w888 w896]
                tunnel: w857 -> [_ w893]
                tunnel: [w887 w892] -> w879
                frame False {
                  n344 = call "Stages Messenger.vi"("Stage Notifier Name"=w888, "Actions"=Stage_Actions."Get Position") -> ("Positions"=w887:dbl[])  [unwired: 10 in, 3 out]
                }
                frame True {
                  n345 = Build Array(w893) -> (w895:dbl[])
                  n346 = call "Stages Messenger.vi"("Stage Notifier Name"=w896, "Actions"=Stage_Actions."MVR", "Setpoint"=w895, "Axis"=bool[] [TRUE], "Exit While Busy?"=FALSE) -> ("Positions"=w892:dbl[])  [unwired: 7 in, 3 out]
                }
              }
              n347 = Select(t=WFDC_Actions."XY Drift" ("x"), s=w855, f=WFDC_Actions."Set Error" ("x")) -> (s? t:f=w852:T10)
              n348 = Index Array(array=w879, index=0) -> (element=→"Z Stage Position":dbl)
            }
            frame "XY Drift" {
              n349 = local read "Cycle Sync XY Correction"() -> (w903:bool)
              n350 = Get Notifier Status(notifier=w907) -> (current notification=w912:T9)  [unwired: 1 in, 4 out]
              n351 = Unbundle By Name(w912) -> ("Cycle Sync"=w911:T7)
              n352 = Equal?(x=w911, y=WFDC_Cycle_Pause."Paused") -> (x = y?=w908:bool)
              n353 = Select(t=w908, s=w903, f=TRUE) -> (s? t:f=w902:bool)
              n354 = And(x="Correct XY Drift", y=w902) -> (x .and. y?=w900:bool)
              n355 = case shown="True" w900 {
                tunnel: w899 -> [_ w941]
                tunnel: w913 -> [_ w928]
                tunnel: w903 -> [_ w917]
                tunnel: [FALSE w916] -> w898
                frame False {
                }
                frame True {
                  n356 = Array Subset(array=w941, index=0, length=2) -> (w920:dbl[])
                  n357 = Negate(x="XY Drift Threshold (pixels)") -> (-x=w924:dbl)
                  n358 = Build Array("Invert X Axis", "Invert Y Axis") -> (w926:bool[])
                  n359 = In Range and Coerce(upper limit="XY Drift Threshold (pixels)", x=w920, lower limit=w924) -> (In Range?=w929:bool[])  [unwired: 1 out]
                  n360 = Not Equal To 0?(x=w920) -> (x != 0?=w921:bool[])
                  n361 = And Array Elements(Boolean array=w929) -> (logical AND=w918:bool)
                  n362 = And Array Elements(Boolean array=w921) -> (logical AND=w919:bool)
                  n363 = case shown="True" "Flip XY Axis" {
                    tunnel: w929 -> [w943 w947]
                    tunnel: [w943 w946] -> w934
                    tunnel: w920 -> [w942 w945]
                    tunnel: [w942 w944] -> w923
                    frame False {
                    }
                    frame True {
                      n364 = Reverse 1D Array(array=w945) -> (reversed array=w944:dbl[])
                      n365 = Reverse 1D Array(array=w947) -> (reversed array=w946:bool[])
                    }
                  }
                  n366 = Compound Arithmetic op=AND(w918, w919, w917) -> (w916:bool)
                  n367 = for {
                    N: 2 -> [_]
                    tunnel: w934 -> [w958] mode=indexing
                    tunnel: [w954] -> w936 mode=indexing
                    tunnel: [w957] -> w937 mode=indexing
                    tunnel: "XY Drift Step (µm)" -> [w949]
                    tunnel: w926 -> [w955] mode=indexing
                    tunnel: w923 -> [w953] mode=indexing
                    tunnel: "XY Drift Threshold (pixels)" -> [w952]
                    n368 = Greater?(x=w953, y=w952) -> (0:w951:bool)
                    n369 = Not(x=w958) -> (.not. x?=w957:bool)
                    n370 = Negate(x=w949) -> (-x=w950:dbl)
                    n371 = Select(t=w949, s=w951, f=w950) -> (s? t:f=w948:dbl)
                    n372 = Negate(x=w948) -> (-x=w956:dbl)
                    n373 = Select(t=w948, s=w955, f=w956) -> (s? t:f=w954:dbl)
                  }
                  n374 = Not(x=w918) -> (.not. x?=→"XY Drift Correction Active":bool)
                  n375 = call "Stages Messenger.vi"("Stage Notifier Name"=w928, "Actions"=Stage_Actions."MVR", "Setpoint"=w936, "Axis"=w937, "Exit While Busy?"=FALSE) -> ()  [unwired: 7 in, 4 out]
                }
              }
              n376 = Select(t=WFDC_Actions."Start Cycle" ("x"), s=w898, f=WFDC_Actions."Get Drift" ("x")) -> (s? t:f=w905:T10)
            }
            frame "Start Cycle" {
              n377 = Get Notifier Status(notifier=w962) -> (current notification=w961:T2)  [unwired: 1 in, 4 out]
              n378 = Unbundle By Name(w961) -> ("Capture?"=w960:bool)
              n379 = case shown="True" w960 {
                tunnel: w963 -> [_ w973]
                frame False {
                }
                frame True {
                  n380 = Get Notifier Status(notifier=w973) -> (notifier out=w974:refnum<notifier>, current notification=w975:T9)  [unwired: 1 in, 3 out]
                  n381 = Bundle By Name(cluster=w975, "Cycle Sync"=WFDC_Cycle_Pause."Resume Requested") -> (w976:T9)
                  n382 = Send Notification(notification=w976, notifier=w974) -> (notifier out=w972:refnum<notifier>)  [unwired: 1 in, 1 out]
                  n383 = while {
                    tunnel: w972 -> [w988]
                    tunnel: [w982] -> w967
                    i -> [w986]
                    stop <- w978 stop-if-true
                    n384 = Wait (ms)(milliseconds to wait=u32 1) -> ()  [unwired: 1 out]
                    n385 = Get Notifier Status(notifier=w988) -> (notifier out=w982:refnum<notifier>, current notification=w983:T9)  [unwired: 1 in, 3 out]
                    n386 = Unbundle By Name(w983) -> ("Cycle Sync"=w981:T7)
                    n387 = Greater?(x=w986, y=4000) -> (0:w984:bool)
                    n388 = Equal?(x=w981, y=WFDC_Cycle_Pause."Resumed") -> (x = y?=w979:bool)
                    n389 = Or(x=w979, y=w984) -> (x .or. y?=w978:bool)
                  }
                  n390 = Get Notifier Status(notifier=w967) -> (notifier out=w971:refnum<notifier>, current notification=w970:T9)  [unwired: 1 in, 3 out]
                  n391 = Bundle By Name(cluster=w970, "Cycle Sync"=WFDC_Cycle_Pause."Pause Requested") -> (w969:T9)
                  n392 = Send Notification(notification=w969, notifier=w971) -> ()  [unwired: 1 in, 2 out]
                }
              }
            }
            frame "Stop DC", "Abort Remote", "Set Error" {
              n393 = Equal?(x=w1001, y=WFDC_Actions."Set Error") -> (x = y?=w994:bool)
              "Error" <- w994
              n394 = And(x=w994, y="Abort Capture If Error") -> (x .and. y?=w998:bool)
              n395 = case shown="True" w994 {
                frame False {
                }
                frame True {
                  n396 = local write "Setup New"(FALSE ("Setup New")) -> ()
                }
              }
              n397 = Get Notifier Status(notifier=w1010) -> (current notification=w1007:T11)  [unwired: 1 in, 4 out]
              n398 = Unbundle By Name(w1007) -> ("Ref Images"=w1009:T3[])
              n399 = Select(t=WFDC_Status."Error" ("WFDC Status"), s=w998, f=WFDC_Status."Idle" ("WFDC Status")) -> (s? t:f=w996:T8)
              n400 = call "IDS Camera Messenger.vi"("Notifier Name"=w1013, "IDS Actions"=IDS_Actions."Abort") -> ()  [unwired: 8 in, 6 out]
              n401 = for {
                tunnel: w1009 -> [w1016] mode=indexing
                n402 = call "IMAQ Dispose"("Image"=w1016) -> ()  [unwired: 5 in, 1 out]
              }
              n403 = Get Notifier Status(notifier=w1003) -> (notifier out=w1004:refnum<notifier>, current notification=w1005:T9)  [unwired: 1 in, 3 out]
              n404 = Bundle By Name(cluster=w1005, "Cycle Sync"=WFDC_Cycle_Pause."Resumed", "WFDC Status"=w996) -> (w1006:T9)
              n405 = Send Notification(notification=w1006, notifier=w1004) -> ()  [unwired: 1 in, 2 out]
              n406 = property on="Main Tab" class="TabCtl (strict)"() -> ("Pages"=w993:refnum<vi>[])  [unwired: 2 in, 2 out]
              n407 = Index Array(array=w993, index=3) -> (element=w991:refnum<vi>)
              n408 = property class="Page"(reference=w991, "PageEnb"=T23."Page Enabled" ("Page Enabled State")) -> ()  [unwired: 1 in, 2 out]
            }
            frame "Exit Loop" {
              n409 = local write "Running"(FALSE ("Running")) -> ()
            }
            frame "Quit" {
              n410 = Release Notifier(notifier=w1028, force destroy? (F)=TRUE) -> ()  [unwired: 1 in, 3 out]
              n411 = Release Notifier(notifier=w1027, force destroy? (F)=TRUE) -> ()  [unwired: 1 in, 3 out]
              n412 = Release Notifier(notifier=w1023) -> ()  [unwired: 2 in, 3 out]
            }
          }
        }
      }
      n413 = while {
        tunnel: w113 -> [w119]
        tunnel: [FALSE] -> w112
        tunnel: w111 -> [w117]
        tunnel: w109 -> [w116]
        stop <- w122 stop-if-true
        # "GUI Control Loop"
        n414 = event shown="[5] \"Abort Remote\": Value Change" {
          selector: _ -> [_ _ _ _ _ _ _ _ _ _ _ _ _]
          dyn-events: _ -> [_ _ _ _ _ _ _ _ _ _ _ _ _]
          timeout: -1 -> [_ _ _ _ _ _ _ _ _ _ _ _ _]
          tunnel: [w123 w135 w136 w149 w155 w161 w170 w173 w182 w187 w194 w198 w225] -> w122
          tunnel: FALSE -> [w123 w135 w136 w149 w155 w161 w170 w173 w182 w187 w194 w198 _]
          tunnel: w119 -> [_ _ _ w145 w150 w156 _ _ _ _ _ _ w231]
          tunnel: w117 -> [_ _ _ _ _ _ w168 _ _ _ _ _ w229]
          tunnel: w116 -> [_ _ _ _ _ _ _ w174 w177 w183 w189 w203 _]
          event Timeout {
            n415 = event-data() -> ()  [unwired: 1 in, 3 out]
          }
          event "Stage Defaults": Value Change {
            n416 = event-data() -> ()  [unwired: 1 in, 1 out]
            n417 = local read "Invert X Axis"() -> (w125:bool)
            n418 = local read "Invert Y Axis"() -> (w126:bool)
            n419 = local read "Flip XY Axis"() -> (w124:bool)
            n420 = Bundle By Name(cluster=T6 {"Flip XY"=FALSE, "Invert X"=FALSE, "Invert Y"=FALSE} ("Default WFDC Stage Settings"), "Flip XY"=w124, "Invert X"=w125, "Invert Y"=w126) -> (w127:T6)
            n421 = control-ref of="This VI"() -> (w134:refnum<vi>)
            n422 = property class="VI"(reference=w134) -> ("Path"=w133:path)  [unwired: 1 in, 2 out]
            n423 = Strip Path(path=w133) -> (stripped path=w132:path)  [unwired: 1 out]
            n424 = Flatten To JSON(anything=w127) -> (JSON string=w129:string)  [unwired: 2 in, 1 out]
            n425 = Build Path(base path=w132, name or relative path="Default WFDC Stage Settings.json") -> (appended path=w130:path)
            n426 = Write to Text File(file (use dialog)=w130, text=w129) -> ()  [unwired: 2 in, 3 out]
          }
          event "Correct XY Drift": Value Change {
            n427 = event-data() -> ("NewVal"=w140:bool)  [unwired: 1 in]
            n428 = Select(t=T16."Enabled" ("Disabled"), s=w140, f=T16."Disabled and Grayed Out") -> (s? t:f=w138:T16)
            n429 = property on="Cycle Sync XY Correction" class="Bool (strict)"("DisabledEnum"=w138) -> ()  [unwired: 2 in, 2 out]
          }
          event "Setup New": Value Change {
            n430 = event-data() -> ("NewVal"=w144:bool)  [unwired: 1 in]
            n431 = Select(t=WFDC_Actions."Setup New DC" ("WFDC Actions"), s=w144, f=WFDC_Actions."Stop DC" ("WFDC Actions")) -> (s? t:f=w142:T10)
            n432 = Get Notifier Status(notifier=w145) -> (notifier out=w147:refnum<notifier>, current notification=w148:T11)  [unwired: 1 in, 3 out]
            n433 = Bundle By Name(cluster=w148, "WFDC Actions"=w142) -> (w146:T11)
            n434 = Send Notification(notification=w146, notifier=w147) -> ()  [unwired: 1 in, 2 out]
          }
          event "Find Focus": Value Change {
            n435 = event-data() -> ()  [unwired: 1 in, 1 out]
            n436 = Get Notifier Status(notifier=w150) -> (notifier out=w153:refnum<notifier>, current notification=w154:T11)  [unwired: 1 in, 3 out]
            n437 = Bundle By Name(cluster=w154, "WFDC Actions"=WFDC_Actions."Remote Start") -> (w152:T11)
            n438 = Send Notification(notification=w152, notifier=w153) -> ()  [unwired: 1 in, 2 out]
          }
          event "Abort Remote": Value Change {
            n439 = event-data() -> ()  [unwired: 1 in, 1 out]
            n440 = Get Notifier Status(notifier=w156) -> (notifier out=w159:refnum<notifier>, current notification=w160:T11)  [unwired: 1 in, 3 out]
            n441 = Bundle By Name(cluster=w160, "WFDC Actions"=WFDC_Actions."Abort Remote") -> (w158:T11)
            n442 = Send Notification(notification=w158, notifier=w159) -> ()  [unwired: 1 in, 2 out]
          }
          event "Cycle Sync XY Correction", "Cycle Sync Z Correction": Value Change {
            n443 = event-data() -> ("NewVal"=w169:bool)  [unwired: 1 in]
            n444 = Get Notifier Status(notifier=w168) -> (notifier out=w163:refnum<notifier>, current notification=w167:T9)  [unwired: 1 in, 3 out]
            n445 = Select(t=WFDC_Cycle_Pause."Pause Requested" ("Cycle Sync"), s=w169, f=WFDC_Cycle_Pause."Resume Requested" ("Cycle Sync")) -> (s? t:f=w164:T7)
            n446 = Bundle By Name(cluster=w167, "Cycle Sync"=w164) -> (w162:T9)
            n447 = Send Notification(notification=w162, notifier=w163) -> ()  [unwired: 1 in, 2 out]
          }
          event "Image Display": Value Change {
            n448 = event-data() -> ("NewVal"=w171:bool)  [unwired: 1 in]
            n449 = call "IDS Camera Messenger.vi"("Notifier Name"=w174, "IDS Actions"=IDS_Actions."Status") -> ("Image Ref"=w172:T3)  [unwired: 8 in, 5 out]
            n450 = call "WFDC Display Cam Image.vi"("Image Ref"=w172, "Display?"=w171) -> ()  [unwired: 14 in]
          }
          event "Exposure Time (ms)": Value Change {
            n451 = event-data() -> ("NewVal"=w178:dbl)  [unwired: 1 in]
            n452 = Bundle By Name(cluster=T19 {"Parameter"=enum."Exposure Time (s)", "Value"=0.0} ("IDS Parameter"), "Parameter"=IDS_Parameter_List."Exposure Time (s)", "Value"=w178) -> (w176:T19)
            n453 = call "IDS Camera Messenger.vi"("Notifier Name"=w177, "IDS Actions"=IDS_Actions."Set Parameter", "IDS Parameter"=w176) -> ()  [unwired: 7 in, 6 out]
          }
          event "Number of Frames", "Image Save Path": Value Change {
            n454 = event-data() -> ()  [unwired: 1 in, 1 out]
            n455 = call "IDS Camera Messenger.vi"("Notifier Name"=w183, "IDS Actions"=IDS_Actions."Record Settings", "# of Frames"="Number of Frames", "File Save Path"="Image Save Path") -> ()  [unwired: 6 in, 6 out]
          }
          event "Live Preview": Value Change {
            # "Set all zeros for full chip"
            n456 = event-data() -> ("NewVal"=w193:bool)  [unwired: 1 in]
            n457 = call "IDS Camera Messenger.vi"("Notifier Name"=w189, "IDS Actions"=IDS_Actions."Set ROI", "ROI Setup"=T20 {"H Offset"=0, "V Offset"=0, "H Width"=0, "V Width"=0}) -> ("Notifier Name (Dup)"=w188:string)  [unwired: 7 in, 5 out]
            n458 = case shown="False" w193 {
              tunnel: [IDS_Actions."Abort" ("IDS Actions") IDS_Actions."Preview" ("IDS Actions")] -> w192
              frame False {
              }
              frame True {
              }
            }
            n459 = call "IDS Camera Messenger.vi"("Notifier Name"=w188, "IDS Actions"=w192) -> ()  [unwired: 8 in, 6 out]
          }
          event "Capture": Value Change {
            # "Set all zeros for full chip"
            n460 = event-data() -> ("NewVal"=w205:bool)  [unwired: 1 in]
            n461 = call "IDS Camera Messenger.vi"("Notifier Name"=w203, "IDS Actions"=IDS_Actions."Set ROI", "ROI Setup"=T20 {"H Offset"=0, "V Offset"=0, "H Width"=0, "V Width"=0}) -> ("Notifier Name (Dup)"=w202:string)  [unwired: 7 in, 5 out]
            n462 = case shown="False" w205 {
              tunnel: [IDS_Actions."Abort" ("IDS Actions") IDS_Actions."Record" ("IDS Actions")] -> w204
              frame False {
              }
              frame True {
              }
            }
            n463 = call "IDS Camera Messenger.vi"("Notifier Name"=w202, "IDS Actions"=w204) -> ("Notifier Name (Dup)"=w199:string)  [unwired: 8 in, 5 out]
            n464 = while {
              tunnel: w199 -> [w222]
              tunnel: [FALSE] -> w197
              stop <- w208 stop-if-true
              n465 = call "IDS Camera Messenger.vi"("Notifier Name"=w222, "IDS Actions"=IDS_Actions."Status") -> ("Running?"=w220:bool, "Image Ref"=w214:T3)  [unwired: 8 in, 4 out]
              n466 = call "IMAQ Read Custom Data"("Key"="Image Data", "Image"=w214) -> ("error out"=w219:errorcluster, "Custom Data Out"=w216:string)  [unwired: 7 in, 1 out]
              n467 = Not(x=w220) -> (.not. x?=w212:bool)
              n468 = Unflatten From JSON(JSON string=w216, type and defaults=T21 {"Frame"=0, "Sensor Height"=0, "Sensor Width"=0, "ROI Height"=0, "ROI Width"=0, "ROI Enable?"=FALSE, "Bit per Pixel"=0} ("IDS IMAQ Key Info"), error in (no error)=w219) -> (value=w218:T21, error out=w213:errorcluster)  [unwired: 4 in]
              n469 = Not(x="Capture") -> (.not. x?=w206:bool)
              n470 = Unbundle By Name(w218) -> ("Frame"=→"Current Frame":u32)
              n471 = Unbundle By Name(w213) -> ("status"=w211:bool)
              n472 = Compound Arithmetic op=OR(w206, w212, w211) -> (w208:bool)
            }
            n473 = local write "Capture"(w197) -> ()
          }
          event "Quit": Value Change {
            n474 = event-data() -> ()  [unwired: 1 in, 1 out]
            n475 = Get Notifier Status(notifier=w231) -> (notifier out=w230:refnum<notifier>, current notification=w233:T11)  [unwired: 1 in, 3 out]
            n476 = Bundle By Name(cluster=w233, "WFDC Actions"=WFDC_Actions."Stop DC") -> (w232:T11)
            n477 = Send Notification(notification=w232, notifier=w230) -> (notifier out=w228:refnum<notifier>)  [unwired: 1 in, 1 out]
            n478 = while {
              tunnel: w229 -> [w255]
              tunnel: w228 -> [w254]
              tunnel: [w254] -> w227
              tunnel: [w245] -> w226
              i -> [w248]
              stop <- w246 stop-if-true
              n479 = Get Notifier Status(notifier=w255) -> (current notification=w253:T9)  [unwired: 1 in, 4 out]
              n480 = Wait (ms)(milliseconds to wait=u32 1) -> ()  [unwired: 1 out]
              n481 = Greater?(x=w248, y=10000) -> (0:w245:bool)
              n482 = Unbundle By Name(w253) -> ("WFDC Status"=w252:T8)
              n483 = Equal?(x=WFDC_Status."Idle", y=w252) -> (x = y?=w249:bool)
              n484 = Or(x=w249, y=w245) -> (x .or. y?=w246:bool)
            }
            n485 = case shown="False" w226 {
              tunnel: w227 -> [w237 _]
              tunnel: [TRUE FALSE] -> w225
              frame False {
                n486 = flat-sequence {
                  tunnel: [w243] -> w238
                  tunnel: w237 -> [w243]
                  frame #0 {
                    n487 = Wait (ms)(milliseconds to wait=u32 20) -> ()  [unwired: 1 out]
                  }
                }
                n488 = Get Notifier Status(notifier=w238) -> (notifier out=w239:refnum<notifier>, current notification=w241:T11)  [unwired: 1 in, 3 out]
                n489 = Bundle By Name(cluster=w241, "WFDC Actions"=WFDC_Actions."Quit") -> (w236:T11)
                n490 = Send Notification(notification=w236, notifier=w239) -> ()  [unwired: 1 in, 2 out]
              }
              frame True {
              }
            }
          }
        }
      }
      n491 = local write "Quit"(w112) -> ()
      n492 = local read "Z Drift Threshold (µm)"() -> (w107:dbl)
      n493 = local read "Z Drift (µm)"() -> (w106:dbl)
      n494 = Absolute Value(x=w106) -> (abs(x)=w104:dbl)
      n495 = Less Or Equal?(x=w104, y=w107) -> (x <= y?=w108:bool)
      n496 = Not(x=w108) -> (.not. x?=w105:bool)
      n497 = local write "Remote Start"(w105) -> ()
      n498 = local write "Running"(w108) -> ()
    }
  }
